vi "plcHMI_rev99.vi"() -> ()   [LabVIEW 2020]
doc: "ADS continuos synchronous write example using base blocks. \n\nThe client writes data synchronously and does wait for the respose from server."
uses:
  Agilent/AgilentTotalCluster.ctl
  Agilent/AgilentControl.ctl
  Agilent/Channel Config.ctl
  <vilib>/Platform/TimedLoop/XDataNode/timing_clust.ctl
  <vilib>/Platform/TimedLoop/XDataNode/nitl_modes.ctl
  <vilib>/Platform/TimedLoop/XDataNode/wakeup.ctl
  <userlib>/Beckhoff-LabVIEW-Interface/_DependsOn/With TypeResolving/Write Sync Single TypeResolved.vi
  <userlib>/Beckhoff-LabVIEW-Interface/_DependsOn/With TypeResolving/Read Sync Single TypeResolved.vi
  <vilib>/Platform/TimedLoop/XDataNode/XDataNode.xnode
  <vilib>/Platform/TimedLoop/XDataNode/XDNodeRunTimeDep.lvlib
panel:
  in  "Tab Control":T1(tab)
  out "error out":errorcluster
  in  "Symbol file path - MUST BE ENTERED\nLoad \"ADS Write AND Read Symbols REV X.X.xml\"":path
  out "bHasMached":bool
  out "Write Status":bool
  out "Read Status":bool
  in  "EXIT HMI":bool caption="STOP HMI\nEXIT HMI"
  out "Internal TwinCAT Handle ID Maps":dbl format="%#_12g"
  in  "802L TDK PSU Voltage Rating (abs(Volts))":i32=12000 min=1 max=50000
  in  "802L TDL PSU Peak Power (J/s)":i32=9000 min=1 max=50000
  in  "HVPS Model":u16(ring) items=["802L-12kV,9000J/s", "802L+50kV,9000J/s", "Other"]
  in  "Voltage Held by PSU":bool
  in  "Log Capacitor Voltage":bool
  in  "Log Temperature Data":bool
  out "Time Since Last Shot":string caption="Elapsed Time Text"
  in  "Duty Cycle":dbl
  in  "Current Control":bool
  out "Expected Voltage":i16
  in  "Dump":bool
  out "EOC":bool
  out "Maximum Test Number Reached":bool
  out "SCR Ready":bool
  in  "START":bool
  in  "STOP":bool
  in  "Hold":bool
  in  "Charge":bool
  in  "Shot":bool
  in  "HV Switch Mode":bool
  in  "CLEAR FAULT":bool
  in  "Manual/Auto":bool=TRUE
  out "Test Interval (Sec)":i32=15 min=0
  in  "Capacitance (uF)":sgl=1e-13 min=0 max=10000 format="%#_6f"
  in  "Target Charge Volt (V) - Min 1500V - TEMPORARY LIMIT 12kV":i32 min=-12000 max=12000 step=1
  out "Estimated Charge Time (seconds)":sgl
  in  "Hold Time Before Shot (seconds)":i16 max=1000
  in  "Max Number of Shots (Test intervals)":i32=1 min=1
  out "Shot Number":i16
  out "Charge Fault":bool=TRUE
  out "Discharge Fault":bool=TRUE
  out "Hold Fault":bool=TRUE
  out "Cap 1 Temp\nExceeded Fault":bool=TRUE
  out "Ambient Temp\nExceeded Fault":bool=TRUE
  out "PSU Fault":bool=TRUE
  out "Control Sys Fault":bool=TRUE
  out "test Running":bool
  out "Test State":string
  out "Cap 1 Voltage":i16
  out "Cap 1 Temperature":i16
  in  "Capacitor Voltage Data Log File Path (.xlsx)":path
  out "Load Temperature":i16
  out "Soft Dump Temp":i16
  out "Ambient Temp":i16
  out "Waveform Chart - Capacitor Voltage (Probe, abs(Volts))":dbl(graph)
  in  "Manual Charge Time (seconds)":sgl max=90
  in  "Reset Test Number":bool
  in  "Cap 1 Fault Temp (Cel)":i16 min=0 max=125
  in  "Capacitor Temperature Data Log File Path (.xlsx)":path
  out "Cap 1 Voltage (HVPS)":i16
  out "Capacitor Voltage":cluster{dbl, dbl}(graph)
  out "EOC":i16(graph)
  out "Soft Exception":bool
  out "PSU HV FB Fault":bool
  out "Charge FB Fault":bool
  out "Softdump FB Fault":bool
  out "SCR FB":i16(graph)
  in  "CH4 Vertical Units":string(combo)="V"
  in  "CH4 Vertical Units/div":dbl=2.0
  in  "Toggle Scope Scale":bool
  in  "CH1 Vertical Units/div":dbl=2.0
  in  "CH1 Vertical Units":string(combo)="V"
  in  "Horizontal Units":enum16{"us", "ms", "s"}(ring)
  in  "Horizontal Units/div":dbl=200.0
  out "Download":bool
  in  "Single":bool
  in  "Stop":bool
  out "Scope Trig":bool
  in  "Agilent Array":T2[](array[typedef])
  out "Process Step":i16
  in  "C:\\HVTest\\Local_Cap_Log_Scope (.xlsx)":path
  out "Stop Loops":bool
  # "CONFIGURATION"
  # "Press STOP HMI instead of\nLabView Abort Execution"
  # "PSU V Rating, Peak Power\nactive when OTHER\nis selected"
  # "INPUT VARIABLES - For TDK Lambda 802L\nMust be written to before START"
  # "FAULT STATUSES"
  # "Set to -1 for automated\nfull charge to setpoint"
  # "MANUAL CONTROLS"
  # "Does not record during \"wait\" and appends to data file. Must be named with .xlsx"
  # "HV Switch Configuration"
  # "Records during \"Test Running.\" Must be named with .xlsx"
  # "Control Sys Faults"
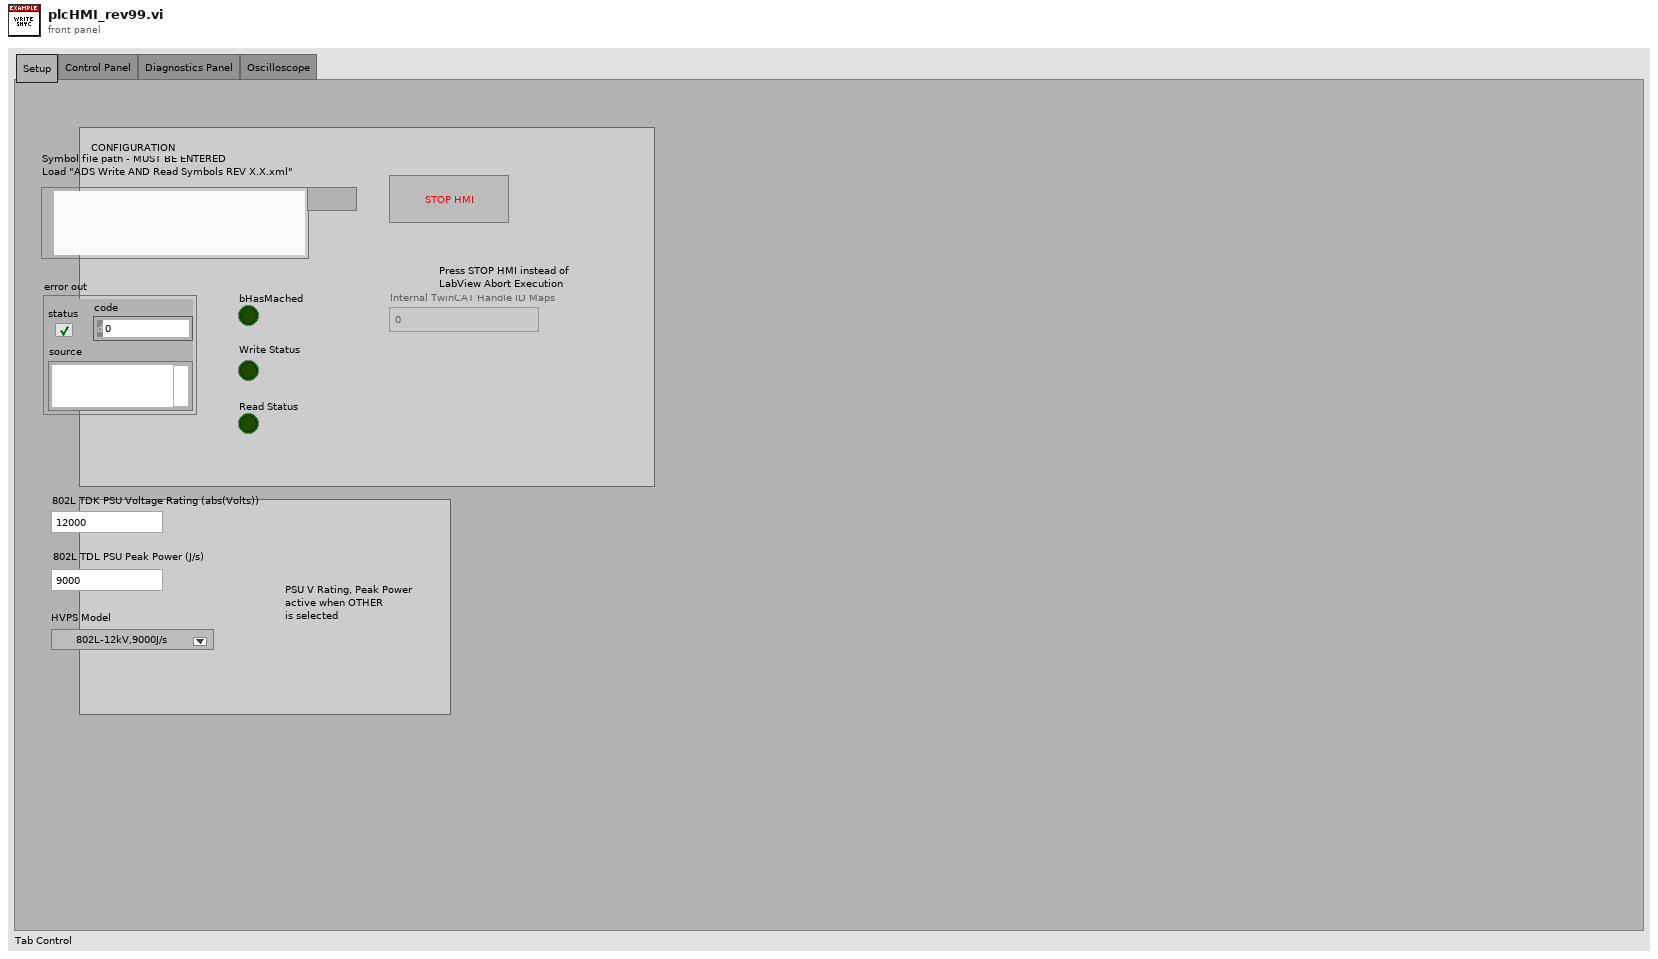
[diagram p1: front panel]
types:
  T1 = enum32{"Setup", "Control Panel", "Diagnostics Panel", "Oscilloscope"}
  T2 = typedef "AgilentTotalCluster.ctl" = cluster{"Agilent Graph":waveform(dbl)[], "Agilent Control":T3, "Agilent Setup Error":errorcluster, "Agilent Present":bool, "Enabled":bool}
  T3 = typedef "AgilentControl.ctl" = cluster{"Trig?":bool, "VISA session":refnum<visa-resource-name>, "Setup to Load":string, "Timeout (ms)":u32, "Desired Samp":enum32{"100", "250", "500", "1000", "2000", "5000", "10000", "20000", "50000", "100000", "200000", "500000", "1000000", "2000000", "4000000", "8000000"}, "Captured Samp":i32, "Desired Channels":T4[]}
  T4 = typedef "Channel Config.ctl" = cluster{"Chan Index":enum16{"Channel1", "Channel2", "Channel3", "Channel4", "MATH"}, "Name":string, "Samples":i32}
  T5 = typedef "XDNodeRunTimeDep.lvlib/timing_clust.ctl" = cluster{"Expected End [f-1]":u64, "Actual End [f-1]":u64, "Finished Late? [f-1]":bool, "Expected End [i-1]":u64, "Actual End [i-1]":u64, "Finished Late? [i-1]":bool, "Expected Start [i]":u64, "Actual Start [i]":u64, "Expected Start [f]":u64, "Actual Start [f]":u64, "Source Name":string, "Structure Name":string, "Period":i64, "Deadline":i64, "Offset":i64, "Start":i64, "Priority":i32, "Timeout":i32, "Mode":T6, "Wakeup Reason":T7, "Error":errorcluster, "Source Type":string, "Secondary Source Type":string, "Global End Time":u64, "Global Start Time":u64, "Frame Duration":u64, "Iteration Duration":u64, "Assigned CPU":i32, "I/O Scan Engine Mode":u32}
  T6 = typedef "XDNodeRunTimeDep.lvlib/nitl_modes.ctl" = enum32{"No Change", "Process missed periods, maintain original phase", "Discard missed periods, maintain original phase", "Process missed periods, ignore original phase", "Discard missed periods, ignore original phase"}
  T7 = typedef "XDNodeRunTimeDep.lvlib/wakeup.ctl" = enum32{"Normal", "Aborted", "Asynchronous wakeup", "Timing source error", "Timed loop error", "Timeout"}
  T8 = cluster{"Agilent Array[0]":T2, "Agilent Array[1]":T2, "Agilent Array[2]":T2, "Agilent Array[3]":T2, "Agilent Array[4]":T2, "Agilent Array[5]":T2, "Agilent Array[6]":T2, "Agilent Array[7]":T2, "Agilent Array[8]":T2}
  T9 = enum32{"100", "250", "500", "1000", "2000", "5000", "10000", "20000", "50000", "100000", "200000", "500000", "1000000", "2000000", "4000000", "8000000"}
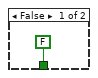
[diagram p2: hidden frame]
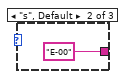
[diagram p5: hidden frame]
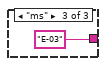
[diagram p6: hidden frame]
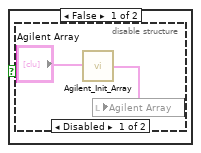
[diagram p7: hidden frame]
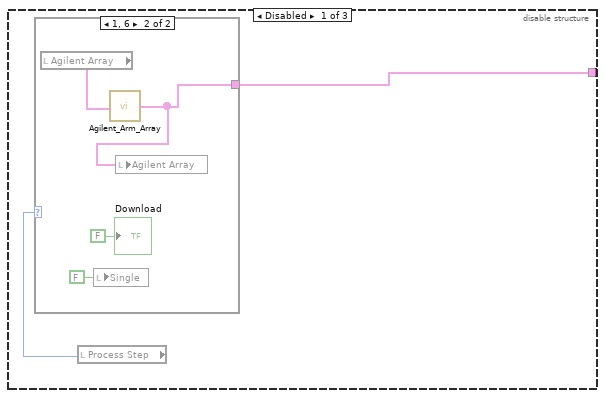
[diagram p11: hidden frame]
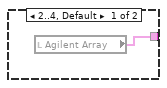
[diagram p12: hidden frame]
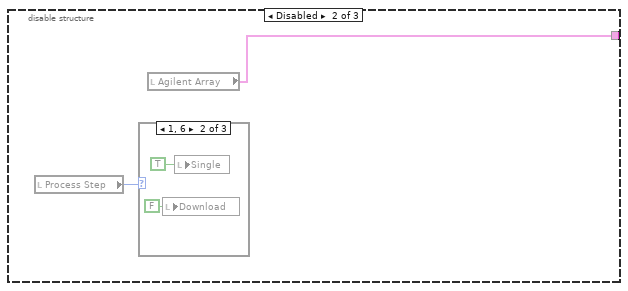
[diagram p13: hidden frame]
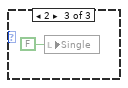
[diagram p15: hidden frame]
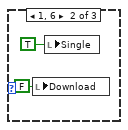
[diagram p17: hidden frame]
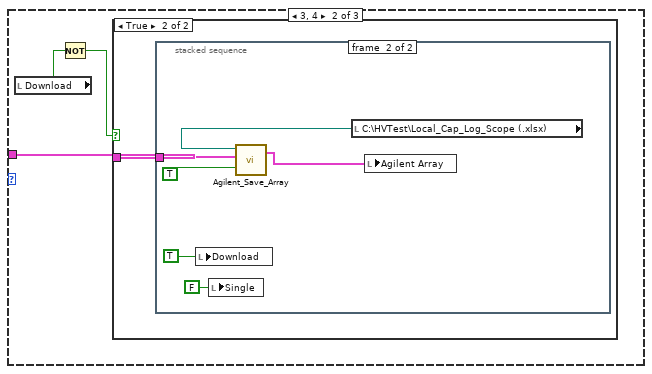
[diagram p19: hidden frame]
diagram:
  w85 = u16 17 items=["SyncLatest"=17, "AsyncLatest"=33] ("WriterMode")
  w154 = u16 33 items=["SyncLatest"=17, "AsyncLatest"=33] ("WriterMode")
  w194 = u16 33 items=["SyncLatest"=17, "AsyncLatest"=33] ("WriterMode")
  w213 = u16 33 items=["SyncLatest"=17, "AsyncLatest"=33] ("WriterMode")
  w232 = u16 33 items=["SyncLatest"=17, "AsyncLatest"=33] ("WriterMode")
  w251 = u16 33 items=["SyncLatest"=17, "AsyncLatest"=33] ("WriterMode")
  w270 = u16 17 items=["SyncLatest"=17, "AsyncLatest"=33] ("WriterMode")
  w289 = u16 17 items=["SyncLatest"=17, "AsyncLatest"=33] ("WriterMode")
  w308 = u16 17 items=["SyncLatest"=17, "AsyncLatest"=33] ("WriterMode")
  w327 = u16 17 items=["SyncLatest"=17, "AsyncLatest"=33] ("WriterMode")
  w346 = u16 17 items=["SyncLatest"=17, "AsyncLatest"=33] ("WriterMode")
  w365 = u16 17 items=["SyncLatest"=17, "AsyncLatest"=33] ("WriterMode")
  w384 = u16 17 items=["SyncLatest"=17, "AsyncLatest"=33] ("WriterMode")
  w399 = u16 17 items=["SyncLatest"=17, "AsyncLatest"=33] ("WriterMode")
  # "Variables/ Control"
  # "Documentation:\nCode separated vertically into two main sections - Write and read\nThey are further separated into BOOL and numeric\nThe OR gates wire all the error lines and the EXIT HMI button to a WHILE LOOP STOP\nThere current delay time on the routine is 100ms\nAll the AND gates connect the typecast resolve lines to the bHasMatched indicator\nThe second and third set of AND gates connect the write statuses to the Write Status indicator\nThe same is done for the read status indicator"
  # "WRITE NUMERICS"
  # "WRITE BOOLS"
  # "Select Symbol N"
  # "Read Initialization"
  # "Release \nTypeResolver"
  # "Release Writer"
  # "Send Request"
  # "Init \nTypeResolver"
  # "Init Writer"
  # "Select Symbol"
  # "Initialization"
  # "Call Release handle block\nat the end, when all nodes\nhave finished their execution"
  # "There must be only one release\nafter every init block.\nRelease block must be called\nalways at the end."
  # "Release"
  # "Symbol Interface"
  n1 = disable-structure shown="Enabled" {
    disable-tunnel: [w405 _] -> w403
    disable-tunnel: [w404 w407] -> w402
    frame Disabled {
      # "Using Symbol Interface"
      n2 = call <userlib>:"Symbol Interface.vi"() -> ("PortInfo"=w404:string, "error out"=w405:errorcluster)  [unwired: 14 in]
    }
    frame Enabled {
      # "Using Symbol File"
      n3 = Path To String(path="Symbol file path - MUST BE ENTERED\nLoad \"ADS Write AND Read Symbols REV X.X.xml\"") -> (string=w407:string)
    }
  }
  n4 = call <userlib>:"Init.vi"("XMLDescription"=w402, "error in (no error)"=w403) -> ("Handle"=w35:u32, "ReadGrpSymbols"=w18:string[], "WriteGrpSymbols"=w23:string[], "error out"=w2:errorcluster)  [unwired: 9 in, 1 out]
  n5 = Index Array(array=w23, index=0) -> (element=w13:string)
  n6 = Index Array(array=w23, index=20) -> (element=w22:string)
  n7 = Index Array(array=w23, index=19) -> (element=w28:string)
  n8 = Index Array(array=w23, index=13) -> (element=w3:string)
  n9 = Index Array(array=w23, index=9) -> (element=w252:string)
  n10 = Index Array(array=w23, index=11) -> (element=w214:string)
  n11 = Index Array(array=w23, index=10) -> (element=w233:string)
  n12 = Index Array(array=w23, index=12) -> (element=w195:string)
  n13 = Index Array(array=w23, index=17) -> (element=w36:string)
  n14 = Index Array(array=w23, index=18) -> (element=w29:string)
  n15 = Index Array(array=w23, index=7) -> (element=w271:string)
  n16 = Index Array(array=w23, index=2) -> (element=w366:string)
  n17 = Index Array(array=w23, index=3) -> (element=w347:string)
  n18 = Index Array(array=w23, index=5) -> (element=w309:string)
  n19 = Index Array(array=w23, index=4) -> (element=w328:string)
  n20 = Index Array(array=w23, index=6) -> (element=w290:string)
  n21 = Index Array(array=w23, index=1) -> (element=w385:string)
  n22 = Index Array(array=w23, index=15) -> (element=w6:string)
  n23 = Index Array(array=w23, index=8) -> (element=w84:string)
  n24 = Index Array(array=w23, index=14) -> (element=w155:string)
  n25 = Index Array(array=w23, index=16) -> (element=w8:string)
  n26 = call <userlib>:"Init Writer.vi"("Handle"=w35, "SymbolName"=w252, "WriterMode"=w251, "error constant"=w2) -> ("Handle"=w250:u32, "SymbolName"=w249:string, "WriterMode"=w248:u16, "WriteHandle"=w247:u32, "error IO"=w246:errorcluster)  [unwired: 7 in]
  n27 = call <userlib>:"Init Writer.vi"("Handle"=w35, "SymbolName"=w214, "WriterMode"=w213, "error constant"=w2) -> ("Handle"=w212:u32, "SymbolName"=w211:string, "WriterMode"=w210:u16, "WriteHandle"=w209:u32, "error IO"=w208:errorcluster)  [unwired: 7 in]
  n28 = call <userlib>:"Init Type.vi"("Handle"=w35, "SymbolName"=w252, "error in"=w2) -> ("Handle"=w245:u32, "TypeHdl"=w244:u32, "error IO"=w243:errorcluster)  [unwired: 7 in, 3 out]
  n29 = call <userlib>:"Init Writer.vi"("Handle"=w35, "SymbolName"=w233, "WriterMode"=w232, "error constant"=w2) -> ("Handle"=w231:u32, "SymbolName"=w230:string, "WriterMode"=w229:u16, "WriteHandle"=w228:u32, "error IO"=w227:errorcluster)  [unwired: 7 in]
  n30 = call <userlib>:"Init Type.vi"("Handle"=w35, "SymbolName"=w214, "error in"=w2) -> ("Handle"=w207:u32, "TypeHdl"=w206:u32, "error IO"=w205:errorcluster)  [unwired: 7 in, 3 out]
  n31 = call <userlib>:"Init Writer.vi"("Handle"=w35, "SymbolName"=w195, "WriterMode"=w194, "error constant"=w2) -> ("Handle"=w193:u32, "SymbolName"=w192:string, "WriterMode"=w191:u16, "WriteHandle"=w190:u32, "error IO"=w189:errorcluster)  [unwired: 7 in]
  n32 = call <userlib>:"Init Type.vi"("Handle"=w35, "SymbolName"=w233, "error in"=w2) -> ("Handle"=w226:u32, "TypeHdl"=w225:u32, "error IO"=w224:errorcluster)  [unwired: 7 in, 3 out]
  n33 = call <userlib>:"Init Type.vi"("Handle"=w35, "SymbolName"=w195, "error in"=w2) -> ("Handle"=w188:u32, "TypeHdl"=w187:u32, "error IO"=w186:errorcluster)  [unwired: 7 in, 3 out]
  n34 = call <userlib>:"Init Writer.vi"("Handle"=w35, "SymbolName"=w271, "WriterMode"=w270, "error constant"=w2) -> ("Handle"=w269:u32, "SymbolName"=w268:string, "WriterMode"=w267:u16, "WriteHandle"=w266:u32, "error IO"=w265:errorcluster)  [unwired: 7 in]
  n35 = call <userlib>:"Init Writer.vi"("Handle"=w35, "SymbolName"=w366, "WriterMode"=w365, "error constant"=w2) -> ("Handle"=w361:u32, "SymbolName"=w360:string, "WriterMode"=w359:u16, "WriteHandle"=w357:u32, "error IO"=w358:errorcluster)  [unwired: 7 in]
  n36 = call <userlib>:"Init Writer.vi"("Handle"=w35, "SymbolName"=w347, "WriterMode"=w346, "error constant"=w2) -> ("Handle"=w345:u32, "SymbolName"=w344:string, "WriterMode"=w343:u16, "WriteHandle"=w342:u32, "error IO"=w341:errorcluster)  [unwired: 7 in]
  n37 = call <userlib>:"Init Writer.vi"("Handle"=w35, "SymbolName"=w309, "WriterMode"=w308, "error constant"=w2) -> ("Handle"=w307:u32, "SymbolName"=w306:string, "WriterMode"=w305:u16, "WriteHandle"=w304:u32, "error IO"=w303:errorcluster)  [unwired: 7 in]
  n38 = call <userlib>:"Init Type.vi"("Handle"=w35, "SymbolName"=w271, "error in"=w2) -> ("Handle"=w264:u32, "TypeHdl"=w263:u32, "error IO"=w262:errorcluster)  [unwired: 7 in, 3 out]
  n39 = call <userlib>:"Init Type.vi"("Handle"=w35, "SymbolName"=w366, "error in"=w2) -> ("Handle"=w350:u32, "TypeHdl"=w349:u32, "error IO"=w348:errorcluster)  [unwired: 7 in, 3 out]
  n40 = call <userlib>:"Init Type.vi"("Handle"=w35, "SymbolName"=w347, "error in"=w2) -> ("Handle"=w340:u32, "TypeHdl"=w339:u32, "error IO"=w338:errorcluster)  [unwired: 7 in, 3 out]
  n41 = call <userlib>:"Init Writer.vi"("Handle"=w35, "SymbolName"=w328, "WriterMode"=w327, "error constant"=w2) -> ("Handle"=w326:u32, "SymbolName"=w325:string, "WriterMode"=w324:u16, "WriteHandle"=w323:u32, "error IO"=w322:errorcluster)  [unwired: 7 in]
  n42 = call <userlib>:"Init Type.vi"("Handle"=w35, "SymbolName"=w309, "error in"=w2) -> ("Handle"=w302:u32, "TypeHdl"=w301:u32, "error IO"=w300:errorcluster)  [unwired: 7 in, 3 out]
  n43 = call <userlib>:"Init Writer.vi"("Handle"=w35, "SymbolName"=w290, "WriterMode"=w289, "error constant"=w2) -> ("Handle"=w288:u32, "SymbolName"=w287:string, "WriterMode"=w286:u16, "WriteHandle"=w285:u32, "error IO"=w284:errorcluster)  [unwired: 7 in]
  n44 = call <userlib>:"Init Type.vi"("Handle"=w35, "SymbolName"=w328, "error in"=w2) -> ("Handle"=w321:u32, "TypeHdl"=w320:u32, "error IO"=w319:errorcluster)  [unwired: 7 in, 3 out]
  n45 = call <userlib>:"Init Type.vi"("Handle"=w35, "SymbolName"=w290, "error in"=w2) -> ("Handle"=w283:u32, "TypeHdl"=w282:u32, "error IO"=w281:errorcluster)  [unwired: 7 in, 3 out]
  n46 = call <userlib>:"Init Writer.vi"("Handle"=w35, "SymbolName"=w385, "WriterMode"=w384, "error constant"=w2) -> ("Handle"=w383:u32, "SymbolName"=w382:string, "WriterMode"=w381:u16, "WriteHandle"=w380:u32, "error IO"=w379:errorcluster)  [unwired: 7 in]
  n47 = call <userlib>:"Init Type.vi"("Handle"=w35, "SymbolName"=w385, "error in"=w2) -> ("Handle"=w378:u32, "TypeHdl"=w377:u32, "error IO"=w376:errorcluster)  [unwired: 7 in, 3 out]
  n48 = call <userlib>:"Init Writer.vi"("Handle"=w35, "SymbolName"=w13, "WriterMode"=w399, "error constant"=w2) -> ("Handle"=w398:u32, "SymbolName"=w397:string, "WriterMode"=w396:u16, "WriteHandle"=w395:u32, "error IO"=w394:errorcluster)  [unwired: 7 in]
  n49 = call <userlib>:"Init Type.vi"("Handle"=w35, "SymbolName"=w13, "error in"=w2) -> ("Handle"=w393:u32, "TypeHdl"=w392:u32, "error IO"=w387:errorcluster)  [unwired: 7 in, 3 out]
  n50 = call <userlib>:"Init Writer.vi"("Handle"=w35, "SymbolName"=w155, "WriterMode"=w154, "error constant"=w2) -> ("Handle"=w150:u32, "SymbolName"=w149:string, "WriterMode"=w148:u16, "WriteHandle"=w140:u32, "error IO"=w147:errorcluster)  [unwired: 7 in]
  n51 = call <userlib>:"Init Type.vi"("Handle"=w35, "SymbolName"=w155, "error in"=w2) -> ("Handle"=w145:u32, "TypeHdl"=w143:u32, "error IO"=w144:errorcluster)  [unwired: 7 in, 3 out]
  n52 = Index Array(array=w18, index=2) -> (element=w136:string)
  n53 = Index Array(array=w18, index=4) -> (element=w132:string)
  n54 = call <userlib>:"Init Writer.vi"("Handle"=w35, "SymbolName"=w84, "WriterMode"=w85, "error constant"=w2) -> ("Handle"=w83:u32, "SymbolName"=w82:string, "WriterMode"=w81:u16, "WriteHandle"=w80:u32, "error IO"=w79:errorcluster)  [unwired: 7 in]
  n55 = Index Array(array=w18, index=1) -> (element=w172:string)
  n56 = Index Array(array=w18, index=21) -> (element=w50:string)
  n57 = Index Array(array=w18, index=22) -> (element=w47:string)
  n58 = call <userlib>:"Init Type.vi"("Handle"=w35, "SymbolName"=w84, "error in"=w2) -> ("Handle"=w78:u32, "TypeHdl"=w77:u32, "error IO"=w76:errorcluster)  [unwired: 7 in, 3 out]
  n59 = Index Array(array=w18, index=0) -> (element=w171:string)
  n60 = Index Array(array=w18, index=3) -> (element=w133:string)
  n61 = Index Array(array=w18, index=20) -> (element=w55:string)
  n62 = Index Array(array=w18, index=23) -> (element=w46:string)
  n63 = Index Array(array=w18, index=16) -> (element=w138:string)
  n64 = Index Array(array=w18, index=24) -> (element=w44:string)
  n65 = Index Array(array=w18, index=11) -> (element=w160:string)
  n66 = Index Array(array=w18, index=10) -> (element=w161:string)
  n67 = Index Array(array=w18, index=17) -> (element=w58:string)
  n68 = Index Array(array=w18, index=18) -> (element=w57:string)
  n69 = Index Array(array=w18, index=13) -> (element=w158:string)
  n70 = Index Array(array=w18, index=12) -> (element=w159:string)
  n71 = Index Array(array=w18, index=15) -> (element=w156:string)
  n72 = Index Array(array=w18, index=19) -> (element=w56:string)
  n73 = Index Array(array=w18, index=26) -> (element=w17:string)
  n74 = Index Array(array=w18, index=5) -> (element=w69:string)
  n75 = Index Array(array=w18, index=6) -> (element=w126:string)
  n76 = Index Array(array=w18, index=9) -> (element=w170:string)
  n77 = Index Array(array=w18, index=14) -> (element=w157:string)
  n78 = Index Array(array=w18, index=8) -> (element=w128:string)
  n79 = Index Array(array=w18, index=25) -> (element=w33:string)
  n80 = Index Array(array=w18, index=7) -> (element=w127:string)
  n81 = node-c288(i64 100 ("Period")) -> (w93:T5)  [unwired: 2 in]
  n82 = timed-loop {
    tunnel: w398 -> [w700]
    tunnel: w397 -> [w699]
    tunnel: w396 -> [w698]
    tunnel: w395 -> [w697]
    tunnel: w393 -> [w929]
    tunnel: w392 -> [w928]
    tunnel: [w695] -> w391
    tunnel: [w694] -> w390
    tunnel: [w927] -> w389
    tunnel: [w926] -> w388
    tunnel: w383 -> [w924]
    tunnel: w382 -> [w923]
    tunnel: w381 -> [w922]
    tunnel: w380 -> [w921]
    tunnel: w378 -> [w919]
    tunnel: w377 -> [w918]
    tunnel: [w916] -> w374
    tunnel: [w915] -> w373
    tunnel: [w914] -> w371
    tunnel: [w913] -> w370
    tunnel: w361 -> [w912]
    tunnel: w360 -> [w911]
    tunnel: w359 -> [w910]
    tunnel: w357 -> [w908]
    tunnel: [w907] -> w356
    tunnel: [w906] -> w355
    tunnel: [w905] -> w352
    tunnel: [w904] -> w351
    tunnel: w350 -> [w903]
    tunnel: w349 -> [w902]
    tunnel: w345 -> [w900]
    tunnel: w344 -> [w899]
    tunnel: w343 -> [w898]
    tunnel: w342 -> [w897]
    tunnel: w340 -> [w895]
    tunnel: w339 -> [w894]
    tunnel: [w892] -> w336
    tunnel: [w891] -> w335
    tunnel: [w890] -> w333
    tunnel: [w889] -> w332
    tunnel: w326 -> [w888]
    tunnel: w325 -> [w887]
    tunnel: w324 -> [w886]
    tunnel: w323 -> [w885]
    tunnel: w321 -> [w883]
    tunnel: w320 -> [w882]
    tunnel: [w880] -> w317
    tunnel: [w879] -> w316
    tunnel: [w878] -> w314
    tunnel: [w877] -> w313
    tunnel: w307 -> [w876]
    tunnel: w306 -> [w875]
    tunnel: w305 -> [w874]
    tunnel: w304 -> [w873]
    tunnel: w302 -> [w871]
    tunnel: w301 -> [w870]
    tunnel: [w868] -> w298
    tunnel: [w867] -> w297
    tunnel: [w866] -> w295
    tunnel: [w865] -> w294
    tunnel: w288 -> [w864]
    tunnel: w287 -> [w863]
    tunnel: w286 -> [w862]
    tunnel: w285 -> [w861]
    tunnel: w283 -> [w859]
    tunnel: w282 -> [w858]
    tunnel: [w856] -> w279
    tunnel: [w855] -> w278
    tunnel: [w854] -> w276
    tunnel: [w853] -> w275
    tunnel: w269 -> [w852]
    tunnel: w268 -> [w851]
    tunnel: w267 -> [w850]
    tunnel: w266 -> [w849]
    tunnel: w264 -> [w847]
    tunnel: w263 -> [w846]
    tunnel: [w844] -> w260
    tunnel: [w843] -> w259
    tunnel: [w842] -> w257
    tunnel: [w841] -> w256
    tunnel: w250 -> [w840]
    tunnel: w249 -> [w839]
    tunnel: w248 -> [w838]
    tunnel: w247 -> [w837]
    tunnel: w245 -> [w835]
    tunnel: w244 -> [w834]
    tunnel: [w832] -> w241
    tunnel: [w831] -> w240
    tunnel: [w830] -> w238
    tunnel: [w829] -> w237
    tunnel: w231 -> [w828]
    tunnel: w230 -> [w827]
    tunnel: w229 -> [w826]
    tunnel: w228 -> [w825]
    tunnel: w226 -> [w823]
    tunnel: w225 -> [w822]
    tunnel: [w820] -> w222
    tunnel: [w819] -> w221
    tunnel: [w818] -> w219
    tunnel: [w817] -> w218
    tunnel: w212 -> [w816]
    tunnel: w211 -> [w815]
    tunnel: w210 -> [w814]
    tunnel: w209 -> [w813]
    tunnel: w207 -> [w811]
    tunnel: w206 -> [w810]
    tunnel: [w808] -> w203
    tunnel: [w807] -> w202
    tunnel: [w806] -> w200
    tunnel: [w805] -> w199
    tunnel: w193 -> [w804]
    tunnel: w192 -> [w803]
    tunnel: w191 -> [w802]
    tunnel: w190 -> [w801]
    tunnel: w188 -> [w799]
    tunnel: w187 -> [w798]
    tunnel: [w796] -> w184
    tunnel: [w795] -> w183
    tunnel: [w794] -> w181
    tunnel: [w793] -> w180
    tunnel: w172 -> [w792]
    tunnel: w171 -> [w791]
    tunnel: w170 -> [w790]
    tunnel: [w789] -> w121
    tunnel: w161 -> [w788]
    tunnel: w160 -> [w787]
    tunnel: w159 -> [w786]
    tunnel: w158 -> [w785]
    tunnel: w157 -> [w784]
    tunnel: w156 -> [w783]
    tunnel: [w782] -> w90
    tunnel: [w781] -> w120
    tunnel: [w780] -> w119
    tunnel: [w779] -> w118
    tunnel: [w778] -> w117
    tunnel: [w723] -> w116
    tunnel: [w721] -> w115
    shift-right: [w626] -> w401
    shift-left: w394 -> [w696]
    shift-right: [w625] -> w400
    shift-left: w387 -> [w925]
    shift-right: [w623] -> w372
    shift-left: w379 -> [w920]
    shift-right: [w622] -> w369
    shift-left: w376 -> [w917]
    shift-right: [w620] -> w354
    shift-left: w358 -> [w909]
    shift-right: [w619] -> w353
    shift-left: w348 -> [w901]
    shift-right: [w617] -> w334
    shift-left: w341 -> [w896]
    shift-right: [w616] -> w331
    shift-left: w338 -> [w893]
    shift-right: [w614] -> w315
    shift-left: w322 -> [w884]
    shift-right: [w613] -> w312
    shift-left: w319 -> [w881]
    shift-right: [w611] -> w296
    shift-left: w303 -> [w872]
    shift-right: [w610] -> w293
    shift-left: w300 -> [w869]
    shift-right: [w608] -> w277
    shift-left: w284 -> [w860]
    shift-right: [w607] -> w274
    shift-left: w281 -> [w857]
    shift-right: [w605] -> w258
    shift-left: w265 -> [w848]
    shift-right: [w604] -> w255
    shift-left: w262 -> [w845]
    shift-right: [w603] -> w239
    shift-left: w246 -> [w836]
    shift-right: [w602] -> w236
    shift-left: w243 -> [w833]
    shift-right: [w600] -> w220
    shift-left: w227 -> [w824]
    shift-right: [w599] -> w217
    shift-left: w224 -> [w821]
    shift-right: [w597] -> w201
    shift-left: w208 -> [w812]
    shift-right: [w596] -> w198
    shift-left: w205 -> [w809]
    shift-right: [w594] -> w182
    shift-left: w189 -> [w800]
    shift-right: [w593] -> w179
    shift-left: w186 -> [w797]
    tunnel: w150 -> [w763]
    tunnel: w149 -> [w762]
    tunnel: w148 -> [w761]
    tunnel: [w759] -> w12
    tunnel: [w758] -> w146
    tunnel: w145 -> [w757]
    tunnel: w143 -> [w755]
    tunnel: [w754] -> w142
    tunnel: [w753] -> w141
    tunnel: w140 -> [w752]
    tunnel: w138 -> [w751]
    tunnel: [w722] -> w114
    tunnel: [w745] -> w123
    tunnel: w2 -> [w744]
    tunnel: [w742] -> w122
    tunnel: w136 -> [w741]
    tunnel: w133 -> [w737]
    tunnel: w132 -> [w736]
    tunnel: [w727] -> w124
    tunnel: [w726] -> w125
    tunnel: w128 -> [w720]
    tunnel: w127 -> [w719]
    tunnel: w126 -> [w718]
    tunnel: [w705] -> w66
    tunnel: [w704] -> w65
    tunnel: [w703] -> w64
    timing: w93 -> [_]
    timing-out: [_] -> w92
    tunnel: w35 -> [w693]
    tunnel: [w591] -> w68
    tunnel: w83 -> [w586]
    tunnel: w82 -> [w585]
    tunnel: w81 -> [w584]
    tunnel: w80 -> [w583]
    tunnel: w78 -> [w581]
    tunnel: w77 -> [w580]
    tunnel: [w577] -> w75
    tunnel: [w576] -> w74
    tunnel: [w575] -> w73
    tunnel: [w574] -> w72
    tunnel: [w567] -> w67
    tunnel: w69 -> [w563]
    tunnel: [w562] -> w63
    tunnel: w58 -> [w559]
    tunnel: w57 -> [w554]
    tunnel: w56 -> [w553]
    tunnel: w55 -> [w552]
    tunnel: [w549] -> w54
    tunnel: [w547] -> w53
    tunnel: [w542] -> w52
    tunnel: [w541] -> w39
    tunnel: w50 -> [w539]
    tunnel: w47 -> [w514]
    tunnel: w46 -> [w513]
    tunnel: w44 -> [w506]
    tunnel: [w502] -> w43
    tunnel: [w501] -> w42
    tunnel: [w500] -> w41
    tunnel: [w499] -> w40
    tunnel: w36 -> [w498]
    tunnel: w35 -> [w417]
    tunnel: w2 -> [w497]
    tunnel: [w494] -> w27
    tunnel: [w493] -> _
    tunnel: w33 -> [w489]
    tunnel: [w485] -> w32
    tunnel: w29 -> [w484]
    tunnel: w28 -> [w483]
    tunnel: w2 -> [w461]
    tunnel: [w478] -> w26
    tunnel: [w477] -> w25
    tunnel: w22 -> [w465]
    tunnel: [w460] -> w21
    tunnel: w17 -> [w447]
    tunnel: [w445] -> w16
    shift-right: [w443] -> w15
    shift-left: w147 -> [w760]
    shift-right: [w442] -> w14
    shift-left: w144 -> [w756]
    tunnel: w2 -> [w435]
    tunnel: [w432] -> w7
    shift-right: [w440] -> w10
    shift-left: w79 -> [w582]
    shift-right: [w439] -> w9
    shift-left: w76 -> [w579]
    tunnel: w8 -> [w434]
    tunnel: w6 -> [w427]
    tunnel: w2 -> [w426]
    tunnel: [w425] -> w5
    tunnel: w3 -> [w418]
    tunnel: w2 -> [w416]
    tunnel: [w415] -> w1
    stop <- w410 stop-if-true
    # "Stop Loop on Error (OR gates)"
    # "Error Stop Loop AND"
    # "Typecast Match AND"
    # "Write Status AND"
    # "READ BOOLS"
    # "READ NUMERICS"
    # "STOP HMI via error or EXIT button"
    # "Check Read status and\nthen convert Variant \nto LabVIEW type (AND gates)"
    # "Sync Read Single"
    n83 = node-c288() -> (w592:errorcluster)  [unwired: 1 in]
    n84 = disable-structure shown="Enabled" {
      frame Enabled {
        n85 = flat-sequence {
          tunnel: [w1061] -> w1005
          tunnel: w1005 -> [w1080]
          frame #0 {
            n86 = disable-structure shown="Enabled" {
              frame Enabled {
                n87 = feedback #1(TRUE) -> (w1007:bool)
                n88 = And(x=TRUE, y=w1007) -> (x .and. y?=w1010:bool)
                n89 = case shown="True" w1010 {
                  tunnel: [FALSE FALSE] -> w1008
                  frame False {
                  }
                  frame True {
                    n90 = local read "Agilent Array"() -> (w1013:T2[])
                    n91 = call "Agilent_Init_Array.vi"("Agilent Array In"=w1013) -> ("Agilent Array Out"=w1014:T2[])
                    n92 = call "Agilent_Arm_Array.vi"("Agilent Array In"=w1014) -> ("Agilent Array Out"=w1012:T2[])
                    n93 = local write "Agilent Array"(w1012) -> ()
                  }
                }
                n94 = feedback-in #1(w1008) -> ()
              }
              frame Disabled {
              }
            }
          }
          frame #1 {
            n95 = case shown="True" "Toggle Scope Scale" {
              frame False {
              }
              frame True {
                n96 = Number To Decimal String(number="CH4 Vertical Units/div") -> (decimal integer string=w1020:string)  [unwired: 1 in]
                n97 = Number To Decimal String(number="Horizontal Units/div") -> (decimal integer string=w1028:string)  [unwired: 1 in]
                n98 = Number To Decimal String(number="CH1 Vertical Units/div") -> (decimal integer string=w1026:string)  [unwired: 1 in]
                n99 = case shown="\"us\"" "Horizontal Units" {
                  tunnel: ["E-06" "E-00" "E-03"] -> w1037
                  frame "us" {
                  }
                  frame "s", Default {
                  }
                  frame "ms" {
                  }
                }
                n100 = Concatenate Strings(":CHAN4:SCAL " ("write buffer"), w1020, "CH4 Vertical Units") -> (w1019:string)
                n101 = Concatenate Strings(":CHAN1:SCAL " ("write buffer"), w1026, "CH1 Vertical Units") -> (w1033:string)
                n102 = Concatenate Strings(":TIM:SCAL " ("write buffer"), w1028, w1037) -> (w1036:string)
                n103 = VISA Open(VISA resource name=refnum<visa-resource-name> "HV_Test_Scope") -> (VISA resource name=w1031:refnum<visa-resource-name>, error out=w1032:errorcluster)  [unwired: 4 in]
                n104 = VISA Write(VISA resource name=w1031, write buffer=w1036, error in (no error)=w1032) -> (VISA resource name out=w1040:refnum<visa-resource-name>, error out=w1039:errorcluster)  [unwired: 1 out]
                n105 = VISA Write(VISA resource name=w1040, write buffer=w1033, error in (no error)=w1039) -> (VISA resource name out=w1025:refnum<visa-resource-name>, error out=w1023:errorcluster)  [unwired: 1 out]
                n106 = VISA Write(VISA resource name=w1025, write buffer=w1019, error in (no error)=w1023) -> (VISA resource name out=w1024:refnum<visa-resource-name>, error out=w1022:errorcluster)  [unwired: 1 out]
                n107 = VISA Close(VISA resource name=w1024, error in (no error)=w1022) -> ()  [unwired: 1 out]
              }
            }
          }
          frame #2 {
            n108 = disable-structure shown="Enabled" {
              frame Enabled {
                n109 = case shown="True" "Stop" {
                  frame False {
                    n110 = disable-structure shown="Disabled" {
                      frame Disabled {
                        n111 = call "Agilent_Init_Array.vi"("Agilent Array In"="Agilent Array") -> ("Agilent Array Out"=w1047:T2[])
                        n112 = local write "Agilent Array"(w1047) -> ()
                      }
                      frame Enabled {
                      }
                    }
                  }
                  frame True {
                    n113 = VISA Open(VISA resource name=refnum<visa-resource-name> "HV_Test_Scope") -> (VISA resource name=w1053:refnum<visa-resource-name>, error out=w1054:errorcluster)  [unwired: 4 in]
                    n114 = VISA Write(VISA resource name=w1053, write buffer=":STOP", error in (no error)=w1054) -> (VISA resource name out=w1051:refnum<visa-resource-name>, error out=w1052:errorcluster)  [unwired: 1 out]
                    n115 = VISA Close(VISA resource name=w1051, error in (no error)=w1052) -> ()  [unwired: 1 out]
                  }
                }
              }
              frame Disabled {
              }
            }
            n116 = case shown="True" "Single" {
              frame False {
              }
              frame True {
                n117 = VISA Open(VISA resource name=refnum<visa-resource-name> "HV_Test_Scope") -> (VISA resource name=w1059:refnum<visa-resource-name>, error out=w1060:errorcluster)  [unwired: 4 in]
                n118 = VISA Write(VISA resource name=w1059, write buffer=":SINGLE", error in (no error)=w1060) -> (VISA resource name out=w1057:refnum<visa-resource-name>, error out=w1058:errorcluster)  [unwired: 1 out]
                n119 = VISA Close(VISA resource name=w1057, error in (no error)=w1058) -> ()  [unwired: 1 out]
              }
            }
          }
          frame #3 {
            n120 = disable-structure shown="Enabled" {
              disable-tunnel: [w1063 w1070 w1075] -> w1061
              frame Disabled {
                n121 = local read "Process Step"() -> (w1062:i16)
                n122 = case shown="1, 6" w1062 {
                  tunnel: [w1064 w1068] -> w1063
                  frame 2..4, Default {
                    n123 = local read "Agilent Array"() -> (w1064:T2[])
                  }
                  frame 1, 6 {
                    n124 = local read "Agilent Array"() -> (w1065:T2[])
                    n125 = local write "Single"(FALSE ("Single")) -> ()
                    n126 = call "Agilent_Arm_Array.vi"("Agilent Array In"=w1065) -> ("Agilent Array Out"=w1068:T2[])
                    n127 = local write "Agilent Array"(w1068) -> ()
                    "Download" <- FALSE ("Downloading")
                  }
                }
              }
              frame Disabled {
                n128 = local read "Process Step"() -> (w1069:i16)
                n129 = case shown="1, 6" w1069 {
                  frame 0, Default {
                  }
                  frame 1, 6 {
                    n130 = local write "Download"(FALSE ("Download")) -> ()
                    n131 = local write "Single"(TRUE ("Single")) -> ()
                  }
                  frame 2 {
                    n132 = local write "Single"(FALSE ("Single")) -> ()
                  }
                }
                n133 = local read "Agilent Array"() -> (w1070:T2[])
              }
              frame Enabled {
                n134 = local read "Process Step"() -> (w1074:i16)
                n135 = case shown="2, 7" w1074 {
                  frame 0, Default {
                  }
                  frame 1, 6 {
                    n136 = local write "Download"(FALSE ("Download")) -> ()
                    n137 = local write "Single"(TRUE ("Single")) -> ()
                  }
                  frame 2, 7 {
                    n138 = local write "Single"(FALSE ("Single")) -> ()
                  }
                }
                n139 = local read "Agilent Array"() -> (w1075:T2[])
              }
            }
          }
          frame #4 {
            n140 = local read "Process Step"() -> (w1079:i16)
            n141 = case shown="0" w1079 {
              tunnel: w1080 -> [_ w1083 w1096]
              frame Default {
              }
              frame 3, 4 {
                n142 = local read "Download"() -> (w1082:bool)
                n143 = Not(x=w1082) -> (.not. x?=w1081:bool)
                n144 = case shown="True" w1081 {
                  tunnel: w1083 -> [_ w1084]
                  frame False {
                  }
                  frame True {
                    n145 = stacked-sequence {
                      tunnel: w1084 -> [_ w1094]
                      frame #0 {
                        n146 = local read "Agilent Array"() -> (w1088:T2[])
                        n147 = Array To Cluster(array=w1088) -> (cluster=w1087:T8)
                        n148 = Unbundle By Name(w1087) -> ("Agilent Array[0].Agilent Control.Desired Samp"=w1085:T9)
                        n149 = call "GF_SetRecordLengthProperly.vi"("Num Samples"=w1085, "VISA resource name"=refnum<visa-resource-name> "HV_Test_Scope") -> ()  [unwired: 1 in, 2 out]
                      }
                      frame #1 {
                        n150 = local write "Download"(TRUE ("Downloading")) -> ()
                        n151 = local write "Single"(FALSE ("Single")) -> ()
                        n152 = local read "C:\\HVTest\\Local_Cap_Log_Scope (.xlsx)"() -> (w1089:path)
                        n153 = call "Agilent_Save_Array.vi"("Agilent Download"=TRUE, "Agilent Array In"=w1094, "File Path"=w1089) -> ("Agilent Array Out"=w1092:T2[])  [unwired: 1 in, 1 out]
                        n154 = local write "Agilent Array"(w1092) -> ()
                      }
                    }
                  }
                }
              }
              frame 0 {
                n155 = local read "Maximum Test Number Reached"() -> (w1095:bool)
                n156 = case shown="True" w1095 {
                  tunnel: w1096 -> [_ w1099]
                  frame False {
                  }
                  frame True {
                    n157 = local read "Download"() -> (w1098:bool)
                    n158 = Not(x=w1098) -> (.not. x?=w1097:bool)
                    n159 = case shown="True" w1097 {
                      tunnel: w1099 -> [_ w1100]
                      frame False {
                      }
                      frame True {
                        n160 = stacked-sequence {
                          tunnel: w1100 -> [_ w1110]
                          frame #0 {
                            n161 = local read "Agilent Array"() -> (w1104:T2[])
                            n162 = Array To Cluster(array=w1104) -> (cluster=w1103:T8)
                            n163 = Unbundle By Name(w1103) -> ("Agilent Array[0].Agilent Control.Desired Samp"=w1101:T9)
                            n164 = call "GF_SetRecordLengthProperly.vi"("Num Samples"=w1101, "VISA resource name"=refnum<visa-resource-name> "HV_Test_Scope") -> ()  [unwired: 1 in, 2 out]
                          }
                          frame #1 {
                            n165 = local write "Download"(TRUE ("Downloading")) -> ()
                            n166 = local write "Single"(FALSE ("Single")) -> ()
                            n167 = call "Agilent_Save_Array.vi"("Agilent Download"=TRUE, "Agilent Array In"=w1110, "File Path"="C:\\HVTest\\Local_Cap_Log_Scope (.xlsx)") -> ("Agilent Array Out"=w1108:T2[])  [unwired: 1 in, 1 out]
                            n168 = local write "Agilent Array"(w1108) -> ()
                          }
                        }
                      }
                    }
                  }
                }
              }
            }
          }
        }
      }
      frame Disabled {
      }
    }
    n169 = To Long Integer(number="Max Number of Shots (Test intervals)") -> (32bit integer=w421:i32)
    n170 = To Variant(anything=w421) -> (Variant=w420:variant)
    n171 = case shown="0, Default" "HVPS Model" {
      tunnel: ["802L TDK PSU Voltage Rating (abs(Volts))" 12000 50000] -> w701
      tunnel: ["802L TDL PSU Peak Power (J/s)" 9000 9000] -> w724
      frame 2 {
      }
      frame 0, Default {
      }
      frame 1 {
      }
    }
    n172 = call-poly <userlib>:"Write TypeResolved.vi"("Handle"=w417, "SymbolName"=w418, "WData"=w420, "error constant"=w416) -> ("Write Status?"=w412:bool, "Has Matched?"=w413:bool, "error out"=w415:errorcluster)  [unwired: 8 in, 1 out]
    n173 = To Single Precision Float(number="Manual Charge Time (seconds)") -> (single precision float=w429:sgl)
    n174 = To Variant(anything=w429) -> (Variant=w428:variant)
    n175 = flat-sequence {
      tunnel: w757 -> [w1208]
      tunnel: w755 -> [w1209]
      tunnel: w756 -> [w1210]
      tunnel: [w1210] -> w767
      tunnel: [w1209] -> w766
      tunnel: [w1208] -> w765
      tunnel: [w1207] -> w764
      tunnel: w724 -> [w1206]
      tunnel: [w1213] -> w442
      tunnel: [w1216] -> w753
      tunnel: [w1215] -> w754
      tunnel: [w1214] -> w444
      tunnel: w767 -> [w1219]
      tunnel: w766 -> [w1218]
      tunnel: w765 -> [w1217]
      tunnel: w764 -> [w1212]
      tunnel: [w1211] -> w650
      frame #0 {
        # "Write Data"
        n176 = To Long Integer(number=w1206) -> (32bit integer=w1205:i32)
        n177 = To Variant(anything=w1205) -> (Variant=w1207:variant)
      }
      frame #1 {
        # "Resolve To TC"
        n178 = call <userlib>:"Resolve To TC Type.vi"("Handle"=w1217, "TypHdl"=w1218, "WData"=w1212, "error in"=w1219) -> ("Handle"=w1215:u32, "TypHdl"=w1216:u32, "bHasMatched"=w1211:bool, "ADSWData"=w1214:variant, "error out"=w1213:errorcluster)  [unwired: 7 in]
      }
    }
    n179 = flat-sequence {
      tunnel: w835 -> [w1358]
      tunnel: w834 -> [w1359]
      tunnel: w833 -> [w1360]
      tunnel: [w1360] -> w969
      tunnel: [w1359] -> w968
      tunnel: [w1358] -> w967
      tunnel: [w1357] -> w966
      tunnel: [w1363] -> w602
      tunnel: [w1366] -> w829
      tunnel: [w1365] -> w830
      tunnel: [w1364] -> w771
      tunnel: w969 -> [w1369]
      tunnel: w968 -> [w1368]
      tunnel: w967 -> [w1367]
      tunnel: w966 -> [w1362]
      tunnel: [w1361] -> w641
      frame #0 {
        # "Write Data"
        n180 = To Single Precision Float(number="Capacitance (uF)") -> (single precision float=w1356:sgl)
        n181 = To Variant(anything=w1356) -> (Variant=w1357:variant)
      }
      frame #1 {
        # "Resolve To TC"
        n182 = call <userlib>:"Resolve To TC Type.vi"("Handle"=w1367, "TypHdl"=w1368, "WData"=w1362, "error in"=w1369) -> ("Handle"=w1365:u32, "TypHdl"=w1366:u32, "bHasMatched"=w1361:bool, "ADSWData"=w1364:variant, "error out"=w1363:errorcluster)  [unwired: 7 in]
      }
    }
    n183 = flat-sequence {
      tunnel: w811 -> [w1328]
      tunnel: w810 -> [w1329]
      tunnel: w809 -> [w1330]
      tunnel: [w1330] -> w961
      tunnel: [w1329] -> w960
      tunnel: [w1328] -> w959
      tunnel: [w1327] -> w958
      tunnel: w701 -> [w1325]
      tunnel: [w1333] -> w596
      tunnel: [w1336] -> w805
      tunnel: [w1335] -> w806
      tunnel: [w1334] -> w769
      tunnel: w961 -> [w1339]
      tunnel: w960 -> [w1338]
      tunnel: w959 -> [w1337]
      tunnel: w958 -> [w1332]
      tunnel: [w1331] -> w645
      frame #0 {
        # "Write Data"
        n184 = To Long Integer(number=w1325) -> (32bit integer=w1326:i32)
        n185 = To Variant(anything=w1326) -> (Variant=w1327:variant)
      }
      frame #1 {
        # "Resolve To TC"
        n186 = call <userlib>:"Resolve To TC Type.vi"("Handle"=w1337, "TypHdl"=w1338, "WData"=w1332, "error in"=w1339) -> ("Handle"=w1335:u32, "TypHdl"=w1336:u32, "bHasMatched"=w1331:bool, "ADSWData"=w1334:variant, "error out"=w1333:errorcluster)  [unwired: 7 in]
      }
    }
    n187 = flat-sequence {
      tunnel: w823 -> [w1343]
      tunnel: w822 -> [w1344]
      tunnel: w821 -> [w1345]
      tunnel: [w1345] -> w965
      tunnel: [w1344] -> w964
      tunnel: [w1343] -> w963
      tunnel: [w1342] -> w962
      tunnel: [w1348] -> w599
      tunnel: [w1351] -> w817
      tunnel: [w1350] -> w818
      tunnel: [w1349] -> w770
      tunnel: w965 -> [w1354]
      tunnel: w964 -> [w1353]
      tunnel: w963 -> [w1352]
      tunnel: w962 -> [w1347]
      tunnel: [w1346] -> w643
      frame #0 {
        # "Write Data"
        n188 = To Long Integer(number="Target Charge Volt (V) - Min 1500V - TEMPORARY LIMIT 12kV") -> (32bit integer=w1341:i32)
        n189 = To Variant(anything=w1341) -> (Variant=w1342:variant)
      }
      frame #1 {
        # "Resolve To TC"
        n190 = call <userlib>:"Resolve To TC Type.vi"("Handle"=w1352, "TypHdl"=w1353, "WData"=w1347, "error in"=w1354) -> ("Handle"=w1350:u32, "TypHdl"=w1351:u32, "bHasMatched"=w1346:bool, "ADSWData"=w1349:variant, "error out"=w1348:errorcluster)  [unwired: 7 in]
      }
    }
    n191 = flat-sequence {
      tunnel: w799 -> [w1313]
      tunnel: w798 -> [w1314]
      tunnel: w797 -> [w1315]
      tunnel: [w1315] -> w957
      tunnel: [w1314] -> w956
      tunnel: [w1313] -> w955
      tunnel: [w1312] -> w954
      tunnel: [w1318] -> w593
      tunnel: [w1321] -> w793
      tunnel: [w1320] -> w794
      tunnel: [w1319] -> w768
      tunnel: w957 -> [w1324]
      tunnel: w956 -> [w1323]
      tunnel: w955 -> [w1322]
      tunnel: w954 -> [w1317]
      tunnel: [w1316] -> w647
      frame #0 {
        # "Write Data"
        n192 = To Word Integer(number="Hold Time Before Shot (seconds)") -> (16bit integer=w1311:i16)
        n193 = To Variant(anything=w1311) -> (Variant=w1312:variant)
      }
      frame #1 {
        # "Resolve To TC"
        n194 = call <userlib>:"Resolve To TC Type.vi"("Handle"=w1322, "TypHdl"=w1323, "WData"=w1317, "error in"=w1324) -> ("Handle"=w1320:u32, "TypHdl"=w1321:u32, "bHasMatched"=w1316:bool, "ADSWData"=w1319:variant, "error out"=w1318:errorcluster)  [unwired: 7 in]
      }
    }
    n195 = To Word Integer(number="Cap 1 Fault Temp (Cel)") -> (16bit integer=w437:i16)
    n196 = flat-sequence {
      tunnel: w847 -> [w1223]
      tunnel: w846 -> [w1224]
      tunnel: w845 -> [w1225]
      tunnel: [w1225] -> w933
      tunnel: [w1224] -> w932
      tunnel: [w1223] -> w931
      tunnel: [w1222] -> w930
      tunnel: [w1228] -> w604
      tunnel: [w1231] -> w841
      tunnel: [w1230] -> w842
      tunnel: [w1229] -> w772
      tunnel: w933 -> [w1234]
      tunnel: w932 -> [w1233]
      tunnel: w931 -> [w1232]
      tunnel: w930 -> [w1227]
      tunnel: [w1226] -> w640
      frame #0 {
        # "Write Data"
        n197 = And(x="CLEAR FAULT", y="CLEAR FAULT") -> (x .and. y?=w1221:bool)
        n198 = To Variant(anything=w1221) -> (Variant=w1222:variant)
      }
      frame #1 {
        # "Resolve To TC"
        n199 = call <userlib>:"Resolve To TC Type.vi"("Handle"=w1232, "TypHdl"=w1233, "WData"=w1227, "error in"=w1234) -> ("Handle"=w1230:u32, "TypHdl"=w1231:u32, "bHasMatched"=w1226:bool, "ADSWData"=w1229:variant, "error out"=w1228:errorcluster)  [unwired: 7 in]
      }
    }
    n200 = flat-sequence {
      tunnel: w895 -> [w1283]
      tunnel: w894 -> [w1284]
      tunnel: w893 -> [w1285]
      tunnel: [w1285] -> w949
      tunnel: [w1284] -> w948
      tunnel: [w1283] -> w947
      tunnel: [w1282] -> w946
      tunnel: [w1288] -> w616
      tunnel: [w1291] -> w889
      tunnel: [w1290] -> w890
      tunnel: [w1289] -> w776
      tunnel: w949 -> [w1294]
      tunnel: w948 -> [w1293]
      tunnel: w947 -> [w1292]
      tunnel: w946 -> [w1287]
      tunnel: [w1286] -> w632
      frame #0 {
        # "Write Data"
        n201 = And(x="Hold", y="Hold") -> (x .and. y?=w1281:bool)
        n202 = To Variant(anything=w1281) -> (Variant=w1282:variant)
      }
      frame #1 {
        # "Resolve To TC"
        n203 = call <userlib>:"Resolve To TC Type.vi"("Handle"=w1292, "TypHdl"=w1293, "WData"=w1287, "error in"=w1294) -> ("Handle"=w1290:u32, "TypHdl"=w1291:u32, "bHasMatched"=w1286:bool, "ADSWData"=w1289:variant, "error out"=w1288:errorcluster)  [unwired: 7 in]
      }
    }
    n204 = flat-sequence {
      tunnel: w871 -> [w1253]
      tunnel: w870 -> [w1254]
      tunnel: w869 -> [w1255]
      tunnel: [w1255] -> w941
      tunnel: [w1254] -> w940
      tunnel: [w1253] -> w939
      tunnel: [w1252] -> w938
      tunnel: [w1258] -> w610
      tunnel: [w1261] -> w865
      tunnel: [w1260] -> w866
      tunnel: [w1259] -> w774
      tunnel: w941 -> [w1264]
      tunnel: w940 -> [w1263]
      tunnel: w939 -> [w1262]
      tunnel: w938 -> [w1257]
      tunnel: [w1256] -> w636
      frame #0 {
        # "Write Data"
        n205 = And(x="Shot", y="Shot") -> (x .and. y?=w1251:bool)
        n206 = To Variant(anything=w1251) -> (Variant=w1252:variant)
      }
      frame #1 {
        # "Resolve To TC"
        n207 = call <userlib>:"Resolve To TC Type.vi"("Handle"=w1262, "TypHdl"=w1263, "WData"=w1257, "error in"=w1264) -> ("Handle"=w1260:u32, "TypHdl"=w1261:u32, "bHasMatched"=w1256:bool, "ADSWData"=w1259:variant, "error out"=w1258:errorcluster)  [unwired: 7 in]
      }
    }
    n208 = flat-sequence {
      tunnel: w903 -> [w1299]
      tunnel: [w1295] -> _
      tunnel: w901 -> [w1300]
      tunnel: [w1300] -> w953
      tunnel: [w1295] -> w952
      tunnel: [w1299] -> w951
      tunnel: [w1298] -> w950
      tunnel: w902 -> [w1295]
      tunnel: [w1303] -> w619
      tunnel: [w1306] -> w905
      tunnel: [w1305] -> w904
      tunnel: [w1304] -> w777
      tunnel: w953 -> [w1309]
      tunnel: w952 -> [w1308]
      tunnel: w951 -> [w1307]
      tunnel: w950 -> [w1302]
      tunnel: [w1301] -> w630
      frame #0 {
        # "Write Data"
        n209 = And(x="Manual/Auto", y="Manual/Auto") -> (x .and. y?=w1297:bool)
        n210 = To Variant(anything=w1297) -> (Variant=w1298:variant)
      }
      frame #1 {
        # "Resolve To TC"
        n211 = call <userlib>:"Resolve To TC Type.vi"("Handle"=w1307, "TypHdl"=w1308, "WData"=w1302, "error in"=w1309) -> ("Handle"=w1305:u32, "TypHdl"=w1306:u32, "bHasMatched"=w1301:bool, "ADSWData"=w1304:variant, "error out"=w1303:errorcluster)  [unwired: 7 in]
      }
    }
    n212 = flat-sequence {
      tunnel: w883 -> [w1268]
      tunnel: w882 -> [w1269]
      tunnel: w881 -> [w1270]
      tunnel: [w1270] -> w945
      tunnel: [w1269] -> w944
      tunnel: [w1268] -> w943
      tunnel: [w1267] -> w942
      tunnel: [w1273] -> w613
      tunnel: [w1276] -> w877
      tunnel: [w1275] -> w878
      tunnel: [w1274] -> w775
      tunnel: w945 -> [w1279]
      tunnel: w944 -> [w1278]
      tunnel: w943 -> [w1277]
      tunnel: w942 -> [w1272]
      tunnel: [w1271] -> w634
      frame #0 {
        # "Write Data"
        n213 = And(x="Charge", y="Charge") -> (x .and. y?=w1266:bool)
        n214 = To Variant(anything=w1266) -> (Variant=w1267:variant)
      }
      frame #1 {
        # "Resolve To TC"
        n215 = call <userlib>:"Resolve To TC Type.vi"("Handle"=w1277, "TypHdl"=w1278, "WData"=w1272, "error in"=w1279) -> ("Handle"=w1275:u32, "TypHdl"=w1276:u32, "bHasMatched"=w1271:bool, "ADSWData"=w1274:variant, "error out"=w1273:errorcluster)  [unwired: 7 in]
      }
    }
    n216 = flat-sequence {
      tunnel: w859 -> [w1238]
      tunnel: w858 -> [w1239]
      tunnel: w857 -> [w1240]
      tunnel: [w1240] -> w937
      tunnel: [w1239] -> w936
      tunnel: [w1238] -> w935
      tunnel: [w1237] -> w934
      tunnel: [w1243] -> w607
      tunnel: [w1246] -> w853
      tunnel: [w1245] -> w854
      tunnel: [w1244] -> w773
      tunnel: w937 -> [w1249]
      tunnel: w936 -> [w1248]
      tunnel: w935 -> [w1247]
      tunnel: w934 -> [w1242]
      tunnel: [w1241] -> w638
      frame #0 {
        # "Write Data"
        n217 = And(x="HV Switch Mode", y="HV Switch Mode") -> (x .and. y?=w1236:bool)
        n218 = To Variant(anything=w1236) -> (Variant=w1237:variant)
      }
      frame #1 {
        # "Resolve To TC"
        n219 = call <userlib>:"Resolve To TC Type.vi"("Handle"=w1247, "TypHdl"=w1248, "WData"=w1242, "error in"=w1249) -> ("Handle"=w1245:u32, "TypHdl"=w1246:u32, "bHasMatched"=w1241:bool, "ADSWData"=w1244:variant, "error out"=w1243:errorcluster)  [unwired: 7 in]
      }
    }
    n220 = flat-sequence {
      tunnel: w919 -> [w1184]
      tunnel: w918 -> [w1185]
      tunnel: w917 -> [w1186]
      tunnel: [w1186] -> w692
      tunnel: [w1185] -> w691
      tunnel: [w1184] -> w690
      tunnel: [w1183] -> w689
      tunnel: w692 -> [w1195]
      tunnel: w691 -> [w1194]
      tunnel: w690 -> [w1193]
      tunnel: w689 -> [w1188]
      tunnel: [w1189] -> w622
      tunnel: [w1192] -> w913
      tunnel: [w1191] -> w914
      tunnel: [w1190] -> w688
      tunnel: [w1187] -> w628
      frame #0 {
        # "Write Data"
        n221 = And(x="STOP", y="STOP") -> (x .and. y?=w1182:bool)
        n222 = To Variant(anything=w1182) -> (Variant=w1183:variant)
      }
      frame #1 {
        # "Resolve To TC"
        n223 = call <userlib>:"Resolve To TC Type.vi"("Handle"=w1193, "TypHdl"=w1194, "WData"=w1188, "error in"=w1195) -> ("Handle"=w1191:u32, "TypHdl"=w1192:u32, "bHasMatched"=w1187:bool, "ADSWData"=w1190:variant, "error out"=w1189:errorcluster)  [unwired: 7 in]
      }
    }
    n224 = flat-sequence {
      tunnel: w581 -> [w1131]
      tunnel: w580 -> [w1127]
      tunnel: w579 -> [w1132]
      tunnel: [w1132] -> w590
      tunnel: [w1127] -> w589
      tunnel: [w1131] -> w588
      tunnel: [w1130] -> w587
      tunnel: [w1135] -> w439
      tunnel: [w1138] -> w574
      tunnel: [w1137] -> w575
      tunnel: [w1136] -> w578
      tunnel: w590 -> [w1141]
      tunnel: w589 -> [w1140]
      tunnel: w588 -> [w1139]
      tunnel: w587 -> [w1134]
      tunnel: [w1133] -> w572
      frame #0 {
        # "Write Data"
        n225 = And(x="Reset Test Number", y="Reset Test Number") -> (x .and. y?=w1129:bool)
        n226 = To Variant(anything=w1129) -> (Variant=w1130:variant)
      }
      frame #1 {
        # "Resolve To TC"
        n227 = call <userlib>:"Resolve To TC Type.vi"("Handle"=w1139, "TypHdl"=w1140, "WData"=w1134, "error in"=w1141) -> ("Handle"=w1137:u32, "TypHdl"=w1138:u32, "bHasMatched"=w1133:bool, "ADSWData"=w1136:variant, "error out"=w1135:errorcluster)  [unwired: 7 in]
      }
    }
    n228 = flat-sequence {
      tunnel: w929 -> [w1150]
      tunnel: w928 -> [w1151]
      tunnel: w925 -> [w1152]
      tunnel: [w1152] -> w687
      tunnel: [w1151] -> w686
      tunnel: [w1150] -> w685
      tunnel: [w1149] -> w684
      tunnel: [w1147] -> _
      tunnel: [w1147] -> w683
      tunnel: w700 -> [w1147]
      tunnel: w699 -> [w1146]
      tunnel: [w1146] -> w682
      tunnel: w698 -> [w1145]
      tunnel: [w1145] -> w681
      tunnel: w697 -> [w1144]
      tunnel: [w1144] -> w680
      tunnel: w696 -> [w1143]
      tunnel: [w1143] -> w679
      tunnel: ["START"] -> w516
      tunnel: w687 -> [w1166]
      tunnel: w686 -> [w1165]
      tunnel: w685 -> [w1164]
      tunnel: w684 -> [w1159]
      tunnel: [w1160] -> w678
      tunnel: [w1163] -> w677
      tunnel: [w1162] -> w676
      tunnel: [w1161] -> w675
      tunnel: [w1158] -> w674
      tunnel: w683 -> [w1157]
      tunnel: [w1157] -> w673
      tunnel: w682 -> [w1156]
      tunnel: [w1156] -> w672
      tunnel: w681 -> [w1155]
      tunnel: [w1155] -> w671
      tunnel: w680 -> [w1154]
      tunnel: [w1154] -> w670
      tunnel: [w1153] -> w669
      tunnel: w679 -> [w1153]
      tunnel: [w1177] -> w652
      tunnel: [w1178] -> w927
      tunnel: [w1179] -> w926
      tunnel: [w1180] -> w625
      tunnel: w678 -> [w1180]
      tunnel: w677 -> [w1179]
      tunnel: w676 -> [w1178]
      tunnel: w675 -> [w1169]
      tunnel: w674 -> [w1177]
      tunnel: w673 -> [w1176]
      tunnel: w672 -> [w1175]
      tunnel: w671 -> [w1174]
      tunnel: w670 -> [w1173]
      tunnel: w669 -> [w1172]
      tunnel: [w1171] -> w695
      tunnel: [w1170] -> w694
      tunnel: [w1168] -> w626
      tunnel: [w1167] -> w667
      frame #0 {
        # "Write Data"
        n229 = And(x="START", y="START") -> (x .and. y?=w1148:bool)
        n230 = To Variant(anything=w1148) -> (Variant=w1149:variant)
      }
      frame #1 {
        # "Resolve To TC"
        n231 = call <userlib>:"Resolve To TC Type.vi"("Handle"=w1164, "TypHdl"=w1165, "WData"=w1159, "error in"=w1166) -> ("Handle"=w1162:u32, "TypHdl"=w1163:u32, "bHasMatched"=w1158:bool, "ADSWData"=w1161:variant, "error out"=w1160:errorcluster)  [unwired: 7 in]
      }
      frame #2 {
        # "Write"
        n232 = call <userlib>:"Send Writer-Request.vi"("Handle"=w1176, "SymbolName"=w1175, "WriterMode"=w1174, "WriteHandle"=w1173, "error constant"=w1172, "ADS Write Data"=w1169) -> ("Handle"=w1171:u32, "WriteHandle"=w1170:u32, "Write status?"=w1167:bool, "error IO"=w1168:errorcluster)  [unwired: 5 in, 1 out]
      }
    }
    n233 = To Variant(anything=w437) -> (Variant=w436:variant)
    n234 = call-poly <userlib>:"Write TypeResolved.vi"("Handle"=w417, "SymbolName"=w427, "WData"=w428, "error constant"=w426) -> ("Write Status?"=w422:bool, "Has Matched?"=w423:bool, "error out"=w425:errorcluster)  [unwired: 8 in, 1 out]
    n235 = call-poly <userlib>:"Write TypeResolved.vi"("Handle"=w417, "SymbolName"=w434, "WData"=w436, "error constant"=w435) -> ("Write Status?"=w431:bool, "Has Matched?"=w433:bool, "error out"=w432:errorcluster)  [unwired: 8 in, 1 out]
    n236 = To Single Precision Float(number="Duty Cycle") -> (single precision float=w475:sgl)
    n237 = And(x="Voltage Held by PSU", y="Voltage Held by PSU") -> (x .and. y?=w464:bool)
    n238 = And(x="Current Control", y="Current Control") -> (x .and. y?=w482:bool)
    n239 = To Variant(anything=w475) -> (Variant=w479:variant)
    n240 = And(x="Dump", y="Dump") -> (x .and. y?=w491:bool)
    n241 = To Variant(anything=w464) -> (Variant=w462:variant)
    n242 = To Variant(anything=w482) -> (Variant=w480:variant)
    n243 = To Variant(anything=w491) -> (Variant=w492:variant)
    n244 = call-poly <userlib>:"Write TypeResolved.vi"("Handle"=w417, "SymbolName"=w465, "WData"=w462, "error constant"=w461) -> ("Write Status?"=w454:bool, "Has Matched?"=w455:bool, "error out"=w460:errorcluster)  [unwired: 8 in, 1 out]
    n245 = flat-sequence {
      tunnel: w792 -> [w1497]
      tunnel: w791 -> [w1495]
      tunnel: w790 -> [w1493]
      tunnel: [w1496] -> w1004
      tunnel: [w1494] -> w1003
      tunnel: [w1492] -> w1002
      tunnel: [w1491] -> w1001
      tunnel: [w1490] -> w1000
      tunnel: [w1489] -> w999
      tunnel: [w1488] -> w998
      tunnel: [w1487] -> w997
      tunnel: [w1486] -> w996
      tunnel: [w1485] -> w995
      tunnel: [w1484] -> w994
      tunnel: w788 -> [w1483]
      tunnel: w787 -> [w1482]
      tunnel: w786 -> [w1481]
      tunnel: w785 -> [w1480]
      tunnel: w784 -> [w1479]
      tunnel: w783 -> [w1478]
      tunnel: [w1477] -> w993
      tunnel: [w1476] -> w992
      tunnel: [w1475] -> w991
      tunnel: [w1474] -> w990
      tunnel: [w1473] -> w989
      tunnel: [w1472] -> w988
      tunnel: [w1471] -> w987
      tunnel: [w1470] -> w986
      tunnel: [w1469] -> w985
      tunnel: [w1468] -> w984
      tunnel: [w1467] -> w983
      tunnel: [w1466] -> w982
      tunnel: [w1465] -> w981
      tunnel: [w1464] -> w980
      tunnel: [w1463] -> w979
      tunnel: [w1462] -> w978
      tunnel: [w1461] -> w977
      tunnel: [w1460] -> w976
      tunnel: [w1459] -> w975
      tunnel: [w1458] -> w974
      tunnel: [w1457] -> w973
      tunnel: [w1456] -> w972
      tunnel: [w1455] -> w971
      tunnel: [w1454] -> w970
      tunnel: w751 -> [w1453]
      tunnel: [w1452] -> w750
      tunnel: [w1451] -> w749
      tunnel: [w1450] -> w748
      tunnel: [w1449] -> w747
      tunnel: [w1448] -> w746
      tunnel: w744 -> [w1371]
      tunnel: [w1447] -> w743
      tunnel: w741 -> [w1446]
      tunnel: [w1445] -> w740
      tunnel: [w1444] -> w739
      tunnel: [w1443] -> w738
      tunnel: w737 -> [w1442]
      tunnel: w736 -> [w1441]
      tunnel: [w1440] -> w735
      tunnel: [w1439] -> w734
      tunnel: [w1438] -> w733
      tunnel: [w1437] -> w732
      tunnel: [w1436] -> w731
      tunnel: [w1435] -> w730
      tunnel: [w1434] -> w729
      tunnel: [w1433] -> w728
      tunnel: w720 -> [w1432]
      tunnel: w719 -> [w1431]
      tunnel: w718 -> [w1430]
      tunnel: [w1429] -> w717
      tunnel: [w1428] -> w716
      tunnel: [w1427] -> w715
      tunnel: [w1426] -> w714
      tunnel: [w1425] -> w713
      tunnel: [w1424] -> w712
      tunnel: [w1423] -> w711
      tunnel: [w1422] -> w710
      tunnel: [w1421] -> w709
      tunnel: [w1420] -> w708
      tunnel: [w1419] -> w707
      tunnel: [w1418] -> w706
      tunnel: [w1372] -> _
      tunnel: w693 -> [w1372]
      tunnel: [w1417] -> w566
      tunnel: [w1416] -> w565
      tunnel: [w1415] -> w564
      tunnel: w563 -> [w1414]
      tunnel: [w1413] -> w560
      tunnel: w559 -> [w1412]
      tunnel: [w1411] -> w558
      tunnel: [w1410] -> w557
      tunnel: [w1409] -> w556
      tunnel: [w1408] -> w555
      tunnel: w554 -> [w1407]
      tunnel: w553 -> [w1406]
      tunnel: w552 -> [w1405]
      tunnel: [w1404] -> w551
      tunnel: [w1403] -> w550
      tunnel: [w1402] -> w548
      tunnel: [w1401] -> w546
      tunnel: [w1400] -> w545
      tunnel: [w1399] -> w544
      tunnel: [w1398] -> w543
      tunnel: [w1397] -> w540
      tunnel: w539 -> [w1396]
      tunnel: [w1395] -> w538
      tunnel: [w1394] -> w537
      tunnel: [w1393] -> w536
      tunnel: w514 -> [w1392]
      tunnel: w513 -> [w1391]
      tunnel: [w1390] -> w512
      tunnel: [w1389] -> w511
      tunnel: [w1388] -> w510
      tunnel: [w1387] -> w509
      tunnel: [w1386] -> w508
      tunnel: [w1385] -> w507
      tunnel: w506 -> [w1384]
      tunnel: [w1383] -> w505
      tunnel: [w1382] -> w504
      tunnel: [w1381] -> w503
      tunnel: w489 -> [w1380]
      tunnel: [w1379] -> w488
      tunnel: [w1378] -> w487
      tunnel: [w1377] -> w486
      tunnel: [w1376] -> w449
      tunnel: [w1375] -> w448
      tunnel: w447 -> [w1374]
      tunnel: [w1373] -> w446
      tunnel: [w1370] -> w441
      tunnel: w1004 -> [w1703]
      tunnel: w1003 -> [w1716]
      tunnel: w1002 -> [_]
      tunnel: w1001 -> [w1702]
      tunnel: w1000 -> [w1701]
      tunnel: w999 -> [w1536]
      tunnel: [w1631] -> w789
      tunnel: w998 -> [w1715]
      tunnel: w997 -> [w1717]
      tunnel: w996 -> [w1719]
      tunnel: w995 -> [w1545]
      tunnel: w994 -> [_]
      tunnel: w993 -> [w1698]
      tunnel: w992 -> [w1713]
      tunnel: w991 -> [w1711]
      tunnel: w990 -> [w1709]
      tunnel: w989 -> [w1707]
      tunnel: w988 -> [w1705]
      tunnel: [w1644] -> w782
      tunnel: w987 -> [w1697]
      tunnel: w986 -> [w1696]
      tunnel: w985 -> [w1695]
      tunnel: w984 -> [w1694]
      tunnel: w983 -> [w1693]
      tunnel: w982 -> [w1692]
      tunnel: w981 -> [_]
      tunnel: w980 -> [w1534]
      tunnel: w979 -> [_]
      tunnel: w978 -> [w1532]
      tunnel: w977 -> [_]
      tunnel: w976 -> [w1530]
      tunnel: w975 -> [_]
      tunnel: w974 -> [w1528]
      tunnel: w973 -> [_]
      tunnel: w972 -> [w1526]
      tunnel: w971 -> [_]
      tunnel: w970 -> [w1524]
      tunnel: [w1646] -> w781
      tunnel: [w1648] -> w780
      tunnel: [w1650] -> w779
      tunnel: [w1652] -> w778
      tunnel: w750 -> [w1522]
      tunnel: w749 -> [w1683]
      tunnel: w748 -> [_]
      tunnel: w747 -> [w1615]
      tunnel: w746 -> [w1679]
      tunnel: [w1635] -> w745
      tunnel: w743 -> [w1682]
      tunnel: [w1633] -> w742
      tunnel: w740 -> [w1681]
      tunnel: w739 -> [w1500]
      tunnel: w738 -> [_]
      tunnel: w735 -> [w1677]
      tunnel: w734 -> [w1676]
      tunnel: w733 -> [w1673]
      tunnel: w732 -> [w1672]
      tunnel: w731 -> [w1671]
      tunnel: w730 -> [w1670]
      tunnel: w729 -> [_]
      tunnel: w728 -> [_]
      tunnel: [w1637] -> w727
      tunnel: [w1639] -> w726
      tunnel: [w1654] -> w723
      tunnel: [w1657] -> w722
      tunnel: [w1656] -> w721
      tunnel: w717 -> [w1668]
      tunnel: w716 -> [w1666]
      tunnel: w715 -> [w1664]
      tunnel: w714 -> [w1540]
      tunnel: w713 -> [w1538]
      tunnel: w712 -> [w1542]
      tunnel: w711 -> [w1663]
      tunnel: w710 -> [w1662]
      tunnel: w709 -> [w1661]
      tunnel: w708 -> [_]
      tunnel: w707 -> [_]
      tunnel: w706 -> [_]
      tunnel: [w1642] -> w705
      tunnel: [w1640] -> w704
      tunnel: [w1629] -> w703
      tunnel: [w1630] -> w411
      tunnel: [w1621] -> w591
      tunnel: [w1623] -> w567
      tunnel: w566 -> [w1544]
      tunnel: w565 -> [w1626]
      tunnel: w564 -> [_]
      tunnel: [w1624] -> w562
      tunnel: w560 -> [w1618]
      tunnel: w558 -> [w1613]
      tunnel: w557 -> [w1610]
      tunnel: w556 -> [w1608]
      tunnel: w555 -> [w1595]
      tunnel: w551 -> [w1520]
      tunnel: w550 -> [w1607]
      tunnel: [w1606] -> w549
      tunnel: w548 -> [w1605]
      tunnel: [w1604] -> w547
      tunnel: w546 -> [w1603]
      tunnel: w545 -> [w1516]
      tunnel: w544 -> [w1602]
      tunnel: w543 -> [w1514]
      tunnel: [w1601] -> w542
      tunnel: [w1600] -> w541
      tunnel: w540 -> [w1518]
      tunnel: [w1599] -> w523
      tunnel: [w1598] -> w521
      tunnel: [w1597] -> w531
      tunnel: w538 -> [w1590]
      tunnel: w537 -> [w1512]
      tunnel: w536 -> [w1593]
      tunnel: [w1592] -> w535
      tunnel: w512 -> [w1586]
      tunnel: w511 -> [w1510]
      tunnel: w510 -> [w1588]
      tunnel: w509 -> [w1587]
      tunnel: w508 -> [w1582]
      tunnel: w507 -> [w1508]
      tunnel: w505 -> [w1568]
      tunnel: w504 -> [w1506]
      tunnel: w503 -> [w1581]
      tunnel: [w1574] -> w502
      tunnel: [w1573] -> w501
      tunnel: [w1572] -> w500
      tunnel: [w1571] -> w499
      tunnel: w488 -> [w1549]
      tunnel: w487 -> [w1566]
      tunnel: w486 -> [w1504]
      tunnel: [w1565] -> w485
      tunnel: w449 -> [w1502]
      tunnel: w448 -> [w1550]
      tunnel: w446 -> [w1498]
      tunnel: [w1546] -> w445
      tunnel: w441 -> [_]
      frame #0 {
        # "Read and Resolve Data."
        # "Read/Resolve Symbol N"
        # "Read Data and Resolve Type"
        n246 = call-poly <userlib>:"Read TypeResolved.vi"("Handle"=w1372, "SymbolName"=w1441, "error constant"=w1371) -> ("Handle"=w1434:u32, "Read Status?"=w1439:bool, "RData"=w1435:variant, "error out"=w1438:errorcluster)  [unwired: 9 in]
        n247 = call-poly <userlib>:"Read TypeResolved.vi"("Handle"=w1372, "SymbolName"=w1442, "error constant"=w1371) -> ("Handle"=w1433:u32, "Read Status?"=w1440:bool, "RData"=w1436:variant, "error out"=w1437:errorcluster)  [unwired: 9 in]
        n248 = call-poly <userlib>:"Read TypeResolved.vi"("Handle"=w1372, "SymbolName"=w1495, "error constant"=w1371) -> ("Handle"=w1485:u32, "Read Status?"=w1487:bool, "RData"=w1491:variant, "error out"=w1496:errorcluster)  [unwired: 9 in]
        n249 = call-poly <userlib>:"Read TypeResolved.vi"("Handle"=w1372, "SymbolName"=w1446, "error constant"=w1371) -> ("Handle"=w1443:u32, "Read Status?"=w1445:bool, "RData"=w1444:variant, "error out"=w1448:errorcluster)  [unwired: 9 in]
        n250 = call-poly <userlib>:"Read TypeResolved.vi"("Handle"=w1372, "SymbolName"=w1497, "error constant"=w1371) -> ("Handle"=w1484:u32, "Read Status?"=w1486:bool, "RData"=w1490:variant, "error out"=w1447:errorcluster)  [unwired: 9 in]
        n251 = call-poly <userlib>:"Read TypeResolved.vi"("Handle"=w1372, "SymbolName"=w1374, "error constant"=w1371) -> ("Read Status?"=w1373:bool, "RData"=w1376:variant, "error out"=w1375:errorcluster)  [unwired: 9 in, 1 out]
        n252 = call-poly <userlib>:"Read TypeResolved.vi"("Handle"=w1372, "SymbolName"=w1493, "error constant"=w1371) -> ("Handle"=w1492:u32, "Read Status?"=w1488:bool, "RData"=w1489:variant, "error out"=w1494:errorcluster)  [unwired: 9 in]
        n253 = call-poly <userlib>:"Read TypeResolved.vi"("Handle"=w1372, "SymbolName"=w1483, "error constant"=w1371) -> ("Handle"=w1465:u32, "Read Status?"=w1472:bool, "RData"=w1464:variant, "error out"=w1471:errorcluster)  [unwired: 9 in]
        n254 = call-poly <userlib>:"Read TypeResolved.vi"("Handle"=w1372, "SymbolName"=w1384, "error constant"=w1371) -> ("Read Status?"=w1383:bool, "RData"=w1382:variant, "error out"=w1381:errorcluster)  [unwired: 9 in, 1 out]
        n255 = call-poly <userlib>:"Read TypeResolved.vi"("Handle"=w1372, "SymbolName"=w1380, "error constant"=w1371) -> ("Read Status?"=w1379:bool, "RData"=w1377:variant, "error out"=w1378:errorcluster)  [unwired: 9 in, 1 out]
        n256 = call-poly <userlib>:"Read TypeResolved.vi"("Handle"=w1372, "SymbolName"=w1481, "error constant"=w1371) -> ("Handle"=w1461:u32, "Read Status?"=w1474:bool, "RData"=w1460:variant, "error out"=w1469:errorcluster)  [unwired: 9 in]
        n257 = call-poly <userlib>:"Read TypeResolved.vi"("Handle"=w1372, "SymbolName"=w1479, "error constant"=w1371) -> ("Handle"=w1457:u32, "Read Status?"=w1476:bool, "RData"=w1456:variant, "error out"=w1467:errorcluster)  [unwired: 9 in]
        n258 = call-poly <userlib>:"Read TypeResolved.vi"("Handle"=w1372, "SymbolName"=w1396, "error constant"=w1371) -> ("Read Status?"=w1395:bool, "RData"=w1394:variant, "error out"=w1393:errorcluster)  [unwired: 9 in, 1 out]
        n259 = call-poly <userlib>:"Read TypeResolved.vi"("Handle"=w1372, "SymbolName"=w1392, "error constant"=w1371) -> ("Read Status?"=w1390:bool, "RData"=w1389:variant, "error out"=w1388:errorcluster)  [unwired: 9 in, 1 out]
        n260 = call-poly <userlib>:"Read TypeResolved.vi"("Handle"=w1372, "SymbolName"=w1391, "error constant"=w1371) -> ("Read Status?"=w1386:bool, "RData"=w1385:variant, "error out"=w1387:errorcluster)  [unwired: 9 in, 1 out]
        n261 = call-poly <userlib>:"Read TypeResolved.vi"("Handle"=w1372, "SymbolName"=w1482, "error constant"=w1371) -> ("Handle"=w1463:u32, "Read Status?"=w1473:bool, "RData"=w1462:variant, "error out"=w1470:errorcluster)  [unwired: 9 in]
        n262 = call-poly <userlib>:"Read TypeResolved.vi"("Handle"=w1372, "SymbolName"=w1480, "error constant"=w1371) -> ("Handle"=w1459:u32, "Read Status?"=w1475:bool, "RData"=w1458:variant, "error out"=w1468:errorcluster)  [unwired: 9 in]
        n263 = call-poly <userlib>:"Read TypeResolved.vi"("Handle"=w1372, "SymbolName"=w1478, "error constant"=w1371) -> ("Handle"=w1455:u32, "Read Status?"=w1477:bool, "RData"=w1454:variant, "error out"=w1466:errorcluster)  [unwired: 9 in]
        n264 = call-poly <userlib>:"Read TypeResolved.vi"("Handle"=w1372, "SymbolName"=w1453, "error constant"=w1371) -> ("Handle"=w1450:u32, "Read Status?"=w1449:bool, "RData"=w1452:variant, "error out"=w1451:errorcluster)  [unwired: 9 in]
        n265 = call-poly <userlib>:"Read TypeResolved.vi"("Handle"=w1372, "SymbolName"=w1412, "error constant"=w1371) -> ("Handle"=w1370:u32, "Read Status?"=w1411:bool, "RData"=w1404:variant, "error out"=w1403:errorcluster)  [unwired: 9 in]
        n266 = call-poly <userlib>:"Read TypeResolved.vi"("Handle"=w1372, "SymbolName"=w1407, "error constant"=w1371) -> ("Read Status?"=w1410:bool, "RData"=w1397:variant, "error out"=w1402:errorcluster)  [unwired: 9 in, 1 out]
        n267 = call-poly <userlib>:"Read TypeResolved.vi"("Handle"=w1372, "SymbolName"=w1405, "error constant"=w1371) -> ("Read Status?"=w1408:bool, "RData"=w1398:variant, "error out"=w1399:errorcluster)  [unwired: 9 in, 1 out]
        n268 = call-poly <userlib>:"Read TypeResolved.vi"("Handle"=w1372, "SymbolName"=w1406, "error constant"=w1371) -> ("Read Status?"=w1409:bool, "RData"=w1400:variant, "error out"=w1401:errorcluster)  [unwired: 9 in, 1 out]
        n269 = call-poly <userlib>:"Read TypeResolved.vi"("Handle"=w1372, "SymbolName"=w1432, "error constant"=w1371) -> ("Handle"=w1420:u32, "Read Status?"=w1429:bool, "RData"=w1425:variant, "error out"=w1421:errorcluster)  [unwired: 9 in]
        n270 = call-poly <userlib>:"Read TypeResolved.vi"("Handle"=w1372, "SymbolName"=w1431, "error constant"=w1371) -> ("Handle"=w1419:u32, "Read Status?"=w1428:bool, "RData"=w1426:variant, "error out"=w1422:errorcluster)  [unwired: 9 in]
        n271 = call-poly <userlib>:"Read TypeResolved.vi"("Handle"=w1372, "SymbolName"=w1414, "error constant"=w1371) -> ("Handle"=w1415:u32, "Read Status?"=w1413:bool, "RData"=w1417:variant, "error out"=w1416:errorcluster)  [unwired: 9 in]
        n272 = call-poly <userlib>:"Read TypeResolved.vi"("Handle"=w1372, "SymbolName"=w1430, "error constant"=w1371) -> ("Handle"=w1418:u32, "Read Status?"=w1427:bool, "RData"=w1424:variant, "error out"=w1423:errorcluster)  [unwired: 9 in]
      }
      frame #1 {
        # "Cast Symbol N to LabVIEW Type"
        # "Variant To Data"
        n273 = To Variant(anything=w1542) -> (Variant=w1541:variant)
        n274 = To Variant(anything=w1514) -> (Variant=w1513:variant)
        n275 = To Variant(anything=w1540) -> (Variant=w1539:variant)
        n276 = To Variant(anything=w1508) -> (Variant=w1507:variant)
        n277 = To Variant(anything=w1510) -> (Variant=w1509:variant)
        n278 = To Variant(anything=w1502) -> (Variant=w1501:variant)
        n279 = To Variant(anything=w1512) -> (Variant=w1511:variant)
        n280 = To Variant(anything=w1504) -> (Variant=w1503:variant)
        n281 = To Variant(anything=w1506) -> (Variant=w1505:variant)
        n282 = To Variant(anything=w1538) -> (Variant=w1537:variant)
        n283 = To Variant(anything=w1522) -> (Variant=w1521:variant)
        n284 = To Variant(anything=w1520) -> (Variant=w1519:variant)
        n285 = To Variant(anything=w1518) -> (Variant=w1517:variant)
        n286 = To Variant(anything=w1532) -> (Variant=w1531:variant)
        n287 = To Variant(anything=w1500) -> (Variant=w1499:variant)
        n288 = To Variant(anything=w1516) -> (Variant=w1515:variant)
        n289 = To Variant(anything=w1536) -> (Variant=w1535:variant)
        n290 = To Variant(anything=w1534) -> (Variant=w1533:variant)
        n291 = To Variant(anything=w1524) -> (Variant=w1523:variant)
        n292 = To Variant(anything=w1544) -> (Variant=w1543:variant)
        n293 = To Variant(anything=w1530) -> (Variant=w1529:variant)
        n294 = To Variant(anything=w1526) -> (Variant=w1525:variant)
        n295 = To Variant(anything=w1528) -> (Variant=w1527:variant)
        n296 = And(x=w1549, y=w1498) -> (x .and. y?=w1548:bool)
        n297 = Variant To Data(error in=w1550, Variant=w1501) -> (data=→"Test Interval (Sec)":i32, error out=w1546:errorcluster)  [unwired: 1 in]
        n298 = And(x=w1568, y=w1548) -> (x .and. y?=w1567:bool)
        n299 = And(x=w1582, y=w1567) -> (x .and. y?=w1583:bool)
        n300 = And(x=w1586, y=w1583) -> (x .and. y?=w1585:bool)
        n301 = And(x=w1590, y=w1585) -> (x .and. y?=w1589:bool)
        n302 = And(x=w1595, y=w1589) -> (x .and. y?=w1594:bool)
        n303 = And(x=w1608, y=w1594) -> (x .and. y?=w1609:bool)
        n304 = And(x=w1610, y=w1609) -> (x .and. y?=w1611:bool)
        n305 = And(x=w1613, y=w1611) -> (x .and. y?=w1612:bool)
        n306 = And(x=w1615, y=w1612) -> (x .and. y?=w1614:bool)
        n307 = And(x=w1698, y=w1614) -> (x .and. y?=w1714:bool)
        n308 = And(x=w1713, y=w1714) -> (x .and. y?=w1712:bool)
        n309 = And(x=w1711, y=w1712) -> (x .and. y?=w1710:bool)
        n310 = And(x=w1709, y=w1710) -> (x .and. y?=w1708:bool)
        n311 = And(x=w1707, y=w1708) -> (x .and. y?=w1706:bool)
        n312 = And(x=w1705, y=w1706) -> (x .and. y?=w1704:bool)
        n313 = And(x=w1715, y=w1704) -> (x .and. y?=w1669:bool)
        n314 = And(x=w1668, y=w1669) -> (x .and. y?=w1667:bool)
        n315 = And(x=w1666, y=w1667) -> (x .and. y?=w1665:bool)
        n316 = And(x=w1664, y=w1665) -> (x .and. y?=w1617:bool)
        n317 = And(x=w1618, y=w1617) -> (x .and. y?=w1616:bool)
        n318 = And(x=w1676, y=w1616) -> (x .and. y?=w1675:bool)
        n319 = And(x=w1677, y=w1675) -> (x .and. y?=w1674:bool)
        n320 = And(x=w1681, y=w1674) -> (x .and. y?=w1680:bool)
        n321 = And(x=w1719, y=w1680) -> (x .and. y?=w1718:bool)
        n322 = Variant To Data(error in=w1626, Variant=w1543) -> (data=→"Cap 1 Voltage (HVPS)":i16, error out=w1624:errorcluster)  [unwired: 1 in]
        n323 = Variant To Data(error in=w1697, Variant=w1533) -> (data=→"Discharge Fault":bool, error out=w1646:errorcluster)  [unwired: 1 in]
        n324 = Variant To Data(error in=w1716, Variant=w1535) -> (data=→"Charge Fault":bool, error out=w1644:errorcluster)  [unwired: 1 in]
        n325 = Variant To Data(error in=w1695, Variant=w1529) -> (data=→"Cap 1 Temp\nExceeded Fault":bool, error out=w1650:errorcluster)  [unwired: 1 in]
        n326 = And(x=w1717, y=w1718) -> (x .and. y?=→"Read Status":bool)
        n327 = Variant To Data(error in=w1696, Variant=w1531) -> (data=→"Hold Fault":bool, error out=w1648:errorcluster)  [unwired: 1 in]
        n328 = Variant To Data(error in=w1663, Variant=w1541) -> (data=→"Load Temperature":i16, error out=w1629:errorcluster)  [unwired: 1 in]
        n329 = Variant To Data(error in=w1694, Variant=w1527) -> (data=→"Ambient Temp\nExceeded Fault":bool, error out=w1652:errorcluster)  [unwired: 1 in]
        n330 = Variant To Data(error in=w1693, Variant=w1525) -> (data=→"PSU Fault":bool, error out=w1654:errorcluster)  [unwired: 1 in]
        n331 = Variant To Data(error in=w1692, Variant=w1523) -> (data=→"Control Sys Fault":bool, error out=w1656:errorcluster)  [unwired: 1 in]
        n332 = Variant To Data(error in=w1683, Variant=w1521) -> (data=→"test Running":bool, error out=w1657:errorcluster)  [unwired: 1 in]
        n333 = Variant To Data(error in=w1661, Variant=w1537) -> (data=→"Ambient Temp":i16, error out=w1642:errorcluster)  [unwired: 1 in]
        n334 = Variant To Data(error in=w1602, Variant=w1513) -> (data=w1597:bool, error out=w1600:errorcluster)  [unwired: 1 in]
        "Soft Exception" <- w1597
        n335 = Variant To Data(error in=w1593, Variant=w1511) -> (data=w1591:bool, error out=w1574:errorcluster)  [unwired: 1 in]
        "EOC" <- w1591
        n336 = Variant To Data(error in=w1662, Variant=w1539) -> (data=→"Soft Dump Temp":i16, error out=w1640:errorcluster)  [unwired: 1 in]
        n337 = Variant To Data(error in=w1607, Variant=w1519) -> (data=w1592:bool, error out=w1606:errorcluster)  [unwired: 1 in]
        "Softdump FB Fault" <- w1592
        n338 = Variant To Data(error in=w1603, Variant=w1515) -> (data=w1598:bool, error out=w1601:errorcluster)  [unwired: 1 in]
        "PSU HV FB Fault" <- w1598
        n339 = Variant To Data(error in=w1588, Variant=w1509) -> (data=w1562:bool, error out=w1573:errorcluster)  [unwired: 1 in]
        "SCR Ready" <- w1562
        n340 = Variant To Data(error in=w1587, Variant=w1507) -> (data=→"Maximum Test Number Reached":bool, error out=w1572:errorcluster)  [unwired: 1 in]
        n341 = Variant To Data(error in=w1605, Variant=w1517) -> (data=w1599:bool, error out=w1604:errorcluster)  [unwired: 1 in]
        "Charge FB Fault" <- w1599
        n342 = Variant To Data(error in=w1566, Variant=w1503) -> (data=w1563:bool, error out=w1565:errorcluster)  [unwired: 1 in]
        "Scope Trig" <- w1563
        n343 = Variant To Data(error in=w1679, Variant=w1499) -> (data=w1564:i16, error out=w1635:errorcluster)  [unwired: 1 in]
        "Process Step" <- w1564
        n344 = Variant To Data(error in=w1673, Variant=w1670) -> (data=→"Cap 1 Temperature":i16, error out=w1639:errorcluster)  [unwired: 1 in]
        n345 = Variant To Data(error in=w1672, Variant=w1671) -> (data=w1580:i16, error out=w1637:errorcluster)  [unwired: 1 in]
        "Cap 1 Voltage" <- w1580
        n346 = Variant To Data(error in=w1581, Variant=w1505) -> (data=w1570:i16, error out=w1571:errorcluster)  [unwired: 1 in]
        "Expected Voltage" <- w1570
        n347 = Variant To Data(error in=w1703, Variant=w1702) -> (data=→"Estimated Charge Time (seconds)":sgl, error out=w1631:errorcluster)  [unwired: 1 in]
        n348 = To Double Precision Float(number=w1580) -> (double precision float=→"Waveform Chart - Capacitor Voltage (Probe, abs(Volts))":dbl)
        n349 = Variant To Data(error in=w1682, Variant=w1701) -> (data=→"Shot Number":i16, error out=w1633:errorcluster)  [unwired: 1 in]
        n350 = case shown="True" "Log Temperature Data" {
          tunnel: [errorcluster {"status"=FALSE, "code"=0, "source"=""} ("error out") w1729] -> w1623
          frame False {
          }
          frame True {
            n351 = local read "Cap 1 Temperature"() -> (w1730:i16)
            n352 = local read "test Running"() -> (w1728:bool)
            n353 = call "Write To Measurement File2"("Signals"=w1730, "Enable"=w1728, "Filename"="Capacitor Temperature Data Log File Path (.xlsx)") -> ("error out"=w1729:errorcluster)  [unwired: 14 in, 2 out]
          }
        }
        n354 = case shown="2" w1564 {
          tunnel: ["Charge" "Current Controlled Charge" "Hold - Ready for Shot" "Hold - Cap Open Circuited" "Shot" "Wait" "Dump" "Error" "Wait"] -> w1678
          tunnel: [TRUE TRUE TRUE TRUE TRUE TRUE FALSE FALSE FALSE] -> w1560
          tunnel: [FALSE ("Reset") FALSE ("Reset") FALSE ("Reset") FALSE ("Reset") TRUE ("Reset") FALSE ("Reset") FALSE ("Reset") TRUE ("Reset") FALSE ("Reset")] -> _
          frame 1 {
          }
          frame 6 {
          }
          frame 2 {
          }
          frame 7 {
          }
          frame 3 {
          }
          frame 4 {
          }
          frame 5 {
          }
          frame 99 {
          }
          frame 0, Default {
          }
        }
        "Test State" <- w1678
        n355 = local write "Scope Trig"(w1563) -> ()
        n356 = local read "Cap 1 Voltage"() -> (w1552:i16)
        n357 = case shown="True" "Log Capacitor Voltage" {
          tunnel: [errorcluster {"status"=FALSE, "code"=0, "source"=""} ("error out") w1726] -> w1621
          tunnel: w1580 -> [_ w1725]
          tunnel: w1560 -> [_ w1724]
          frame False {
          }
          frame True {
            n358 = local read "test Running"() -> (w1721:bool)
            n359 = And(x=w1724, y=w1721) -> (x .and. y?=w1722:bool)
            n360 = call "Write To Measurement File"("Signals"=w1725, "Enable"=w1722, "Filename"="Capacitor Voltage Data Log File Path (.xlsx)") -> ("error out"=w1726:errorcluster)  [unwired: 14 in, 2 out]
          }
        }
        n361 = Not(x=w1591) -> (.not. x?=w1578:bool)
        n362 = To Double Precision Float(number=w1552) -> (double precision float=w1576:dbl)
        n363 = To Double Precision Float(number=w1570) -> (double precision float=w1569:dbl)
        n364 = Boolean To (0,1)(Boolean=w1578) -> (0, 1=→"EOC":i16)
        n365 = Or(x=w1656, y=w1657) -> (x .or. y?=w1655:bool)
        n366 = Or(x=w1654, y=w1655) -> (x .or. y?=w1653:bool)
        n367 = Or(x=w1652, y=w1653) -> (x .or. y?=w1651:bool)
        n368 = Or(x=w1650, y=w1651) -> (x .or. y?=w1649:bool)
        n369 = Or(x=w1648, y=w1649) -> (x .or. y?=w1647:bool)
        n370 = Or(x=w1646, y=w1647) -> (x .or. y?=w1645:bool)
        n371 = Or(x=w1644, y=w1645) -> (x .or. y?=w1643:bool)
        n372 = Or(x=w1642, y=w1643) -> (x .or. y?=w1641:bool)
        n373 = Or(x=w1640, y=w1641) -> (x .or. y?=w1628:bool)
        n374 = Or(x=w1629, y=w1628) -> (x .or. y?=w1622:bool)
        n375 = Boolean To (0,1)(Boolean=w1562) -> (0, 1=→"SCR FB":i16)
        n376 = Bundle(w1576, w1569) -> (→"Capacitor Voltage":cluster{dbl, dbl})  [unwired: 1 in]
        n377 = local write "Process Step"(w1564) -> ()
        n378 = local read "Scope Trig"() -> (w1555:bool)
        n379 = local read "Test Interval (Sec)"() -> (w1558:i32)
        n380 = Not(x=w1555) -> (.not. x?=w1554:bool)
        n381 = call "Elapsed Time"("Time Target (s)"=w1558, "Reset"=w1554) -> ("Elapsed Time Text"=w1557:string)  [unwired: 10 in, 7 out]
        n382 = String Subset(string=w1557, offset (0)=2) -> (substring=→"Time Since Last Shot":string)  [unwired: 1 in]
        n383 = Or(x=w1623, y=w1622) -> (x .or. y?=w1620:bool)
        n384 = Or(x=w1621, y=w1620) -> (x .or. y?=w1619:bool)
        n385 = Or(x=w1639, y=w1619) -> (x .or. y?=w1638:bool)
        n386 = Or(x=w1637, y=w1638) -> (x .or. y?=w1636:bool)
        n387 = Or(x=w1635, y=w1636) -> (x .or. y?=w1634:bool)
        n388 = Or(x=w1633, y=w1634) -> (x .or. y?=w1632:bool)
        n389 = Or(x=w1631, y=w1632) -> (x .or. y?=w1630:bool)
        "Internal TwinCAT Handle ID Maps" <- w1545
      }
    }
    n390 = call-poly <userlib>:"Write TypeResolved.vi"("Handle"=w417, "SymbolName"=w483, "WData"=w479, "error constant"=w461) -> ("Write Status?"=w453:bool, "Has Matched?"=w456:bool, "error out"=w477:errorcluster)  [unwired: 8 in, 1 out]
    n391 = call-poly <userlib>:"Write TypeResolved.vi"("Handle"=w417, "SymbolName"=w484, "WData"=w480, "error constant"=w461) -> ("Write Status?"=w452:bool, "Has Matched?"=w457:bool, "error out"=w478:errorcluster)  [unwired: 8 in, 1 out]
    n392 = call <userlib>:"Send Writer-Request.vi"("Handle"=w924, "SymbolName"=w923, "WriterMode"=w922, "WriteHandle"=w921, "error constant"=w920, "ADS Write Data"=w688) -> ("Handle"=w916:u32, "WriteHandle"=w915:u32, "Write status?"=w666:bool, "error IO"=w623:errorcluster)  [unwired: 5 in, 1 out]
    n393 = call-poly <userlib>:"Write TypeResolved.vi"("Handle"=w417, "SymbolName"=w498, "WData"=w492, "error constant"=w497) -> ("Handle"=w493:u32, "Write Status?"=w451:bool, "Has Matched?"=w459:bool, "error out"=w494:errorcluster)  [unwired: 8 in]
    n394 = call <userlib>:"Send Writer-Request.vi"("Handle"=w763, "SymbolName"=w762, "WriterMode"=w761, "WriteHandle"=w752, "error constant"=w760, "ADS Write Data"=w444) -> ("Handle"=w759:u32, "WriteHandle"=w758:u32, "Write status?"=w470:bool, "error IO"=w443:errorcluster)  [unwired: 5 in, 1 out]
    n395 = call <userlib>:"Send Writer-Request.vi"("Handle"=w840, "SymbolName"=w839, "WriterMode"=w838, "WriteHandle"=w837, "error constant"=w836, "ADS Write Data"=w771) -> ("Handle"=w832:u32, "WriteHandle"=w831:u32, "Write status?"=w474:bool, "error IO"=w603:errorcluster)  [unwired: 5 in, 1 out]
    n396 = call <userlib>:"Send Writer-Request.vi"("Handle"=w816, "SymbolName"=w815, "WriterMode"=w814, "WriteHandle"=w813, "error constant"=w812, "ADS Write Data"=w769) -> ("Handle"=w808:u32, "WriteHandle"=w807:u32, "Write status?"=w472:bool, "error IO"=w597:errorcluster)  [unwired: 5 in, 1 out]
    n397 = call <userlib>:"Send Writer-Request.vi"("Handle"=w828, "SymbolName"=w827, "WriterMode"=w826, "WriteHandle"=w825, "error constant"=w824, "ADS Write Data"=w770) -> ("Handle"=w820:u32, "WriteHandle"=w819:u32, "Write status?"=w473:bool, "error IO"=w600:errorcluster)  [unwired: 5 in, 1 out]
    n398 = call <userlib>:"Send Writer-Request.vi"("Handle"=w804, "SymbolName"=w803, "WriterMode"=w802, "WriteHandle"=w801, "error constant"=w800, "ADS Write Data"=w768) -> ("Handle"=w796:u32, "WriteHandle"=w795:u32, "Write status?"=w471:bool, "error IO"=w594:errorcluster)  [unwired: 5 in, 1 out]
    n399 = call <userlib>:"Send Writer-Request.vi"("Handle"=w912, "SymbolName"=w911, "WriterMode"=w910, "WriteHandle"=w908, "error constant"=w909, "ADS Write Data"=w777) -> ("Handle"=w907:u32, "WriteHandle"=w906:u32, "Write status?"=w654:bool, "error IO"=w620:errorcluster)  [unwired: 5 in, 1 out]
    n400 = call <userlib>:"Send Writer-Request.vi"("Handle"=w852, "SymbolName"=w851, "WriterMode"=w850, "WriteHandle"=w849, "error constant"=w848, "ADS Write Data"=w772) -> ("Handle"=w844:u32, "WriteHandle"=w843:u32, "Write status?"=w664:bool, "error IO"=w605:errorcluster)  [unwired: 5 in, 1 out]
    n401 = call <userlib>:"Send Writer-Request.vi"("Handle"=w900, "SymbolName"=w899, "WriterMode"=w898, "WriteHandle"=w897, "error constant"=w896, "ADS Write Data"=w776) -> ("Handle"=w892:u32, "WriteHandle"=w891:u32, "Write status?"=w656:bool, "error IO"=w617:errorcluster)  [unwired: 5 in, 1 out]
    n402 = call <userlib>:"Send Writer-Request.vi"("Handle"=w876, "SymbolName"=w875, "WriterMode"=w874, "WriteHandle"=w873, "error constant"=w872, "ADS Write Data"=w774) -> ("Handle"=w868:u32, "WriteHandle"=w867:u32, "Write status?"=w660:bool, "error IO"=w611:errorcluster)  [unwired: 5 in, 1 out]
    n403 = call <userlib>:"Send Writer-Request.vi"("Handle"=w888, "SymbolName"=w887, "WriterMode"=w886, "WriteHandle"=w885, "error constant"=w884, "ADS Write Data"=w775) -> ("Handle"=w880:u32, "WriteHandle"=w879:u32, "Write status?"=w658:bool, "error IO"=w614:errorcluster)  [unwired: 5 in, 1 out]
    n404 = call <userlib>:"Send Writer-Request.vi"("Handle"=w864, "SymbolName"=w863, "WriterMode"=w862, "WriteHandle"=w861, "error constant"=w860, "ADS Write Data"=w773) -> ("Handle"=w856:u32, "WriteHandle"=w855:u32, "Write status?"=w662:bool, "error IO"=w608:errorcluster)  [unwired: 5 in, 1 out]
    n405 = call <userlib>:"Send Writer-Request.vi"("Handle"=w586, "SymbolName"=w585, "WriterMode"=w584, "WriteHandle"=w583, "error constant"=w582, "ADS Write Data"=w578) -> ("Handle"=w577:u32, "WriteHandle"=w576:u32, "Write status?"=w570:bool, "error IO"=w440:errorcluster)  [unwired: 5 in, 1 out]
    n406 = Compound Arithmetic op=AND(w459, w457, w456, w455) -> (w458:bool)
    n407 = And(x=w433, y=w458) -> (x .and. y?=w495:bool)
    n408 = And(x=w423, y=w495) -> (x .and. y?=w568:bool)
    n409 = And(x=w650, y=w568) -> (x .and. y?=w649:bool)
    n410 = And(x=w413, y=w649) -> (x .and. y?=w648:bool)
    n411 = And(x=w647, y=w648) -> (x .and. y?=w646:bool)
    n412 = And(x=w645, y=w646) -> (x .and. y?=w644:bool)
    n413 = And(x=w643, y=w644) -> (x .and. y?=w642:bool)
    n414 = And(x=w641, y=w642) -> (x .and. y?=w408:bool)
    n415 = And(x=w572, y=w408) -> (x .and. y?=w573:bool)
    n416 = And(x=w640, y=w573) -> (x .and. y?=w639:bool)
    n417 = And(x=w638, y=w639) -> (x .and. y?=w637:bool)
    n418 = And(x=w636, y=w637) -> (x .and. y?=w635:bool)
    n419 = And(x=w634, y=w635) -> (x .and. y?=w633:bool)
    n420 = And(x=w632, y=w633) -> (x .and. y?=w631:bool)
    n421 = And(x=w630, y=w631) -> (x .and. y?=w629:bool)
    n422 = And(x=w628, y=w629) -> (x .and. y?=w627:bool)
    n423 = And(x=w652, y=w627) -> (x .and. y?=→"bHasMached":bool)
    n424 = Compound Arithmetic op=AND(w451, w452, w453, w454) -> (w450:bool)
    n425 = And(x=w431, y=w450) -> (x .and. y?=w496:bool)
    n426 = And(x=w422, y=w496) -> (x .and. y?=w467:bool)
    n427 = Compound Arithmetic op=AND(w474, w473, w472, w471, w412, w470) -> (w469:bool)
    n428 = Not(x=w469) -> (.not. x?=w468:bool)
    n429 = And(x=w468, y=w467) -> (x .and. y?=w466:bool)
    n430 = And(x=w570, y=w466) -> (x .and. y?=w571:bool)
    n431 = And(x=w664, y=w571) -> (x .and. y?=w663:bool)
    n432 = And(x=w662, y=w663) -> (x .and. y?=w661:bool)
    n433 = And(x=w660, y=w661) -> (x .and. y?=w659:bool)
    n434 = And(x=w658, y=w659) -> (x .and. y?=w657:bool)
    n435 = And(x=w656, y=w657) -> (x .and. y?=w655:bool)
    n436 = And(x=w654, y=w655) -> (x .and. y?=w653:bool)
    n437 = And(x=w666, y=w653) -> (x .and. y?=w665:bool)
    n438 = And(x=w667, y=w665) -> (x .and. y?=→"Write Status":bool)
    n439 = feedback #2(TRUE) -> (w518:bool)
    n440 = And(x=w518, y=w521) -> (x .and. y?=w520:bool)
    n441 = feedback #3(TRUE) -> (w528:bool)
    n442 = And(x=w528, y=w531) -> (x .and. y?=w530:bool)
    n443 = feedback #4(TRUE) -> (w532:bool)
    n444 = And(x=w532, y=w535) -> (x .and. y?=w534:bool)
    n445 = feedback #5(TRUE) -> (w524:bool)
    n446 = And(x=w524, y=w523) -> (x .and. y?=w525:bool)
    n447 = case shown="True" w525 {
      tunnel: [w1115 FALSE] -> w515
      tunnel: w516 -> [w1117 _]
      frame False {
        n448 = Or(x=w1117, y=FALSE) -> (x .or. y?=w1115:bool)
      }
      frame True {
        n449 = call "Charge relay error"() -> ()  [unwired: 10 in, 2 out]
      }
    }
    n450 = feedback-in #5(w515) -> ()
    n451 = case shown="True" w520 {
      tunnel: [w1113 FALSE] -> w519
      tunnel: w515 -> [w1111 _]
      frame False {
        n452 = Or(x=w1111, y=FALSE) -> (x .or. y?=w1113:bool)
      }
      frame True {
        n453 = call "PSU HV error"() -> ()  [unwired: 10 in, 2 out]
      }
    }
    n454 = feedback-in #2(w519) -> ()
    n455 = case shown="True" w534 {
      tunnel: [w1124 FALSE] -> w533
      tunnel: w516 -> [w1123 _]
      frame False {
        n456 = Or(x=w1123, y=FALSE) -> (x .or. y?=w1124:bool)
      }
      frame True {
        n457 = call "Softdump error"() -> ()  [unwired: 10 in, 2 out]
      }
    }
    n458 = feedback-in #4(w533) -> ()
    n459 = case shown="True" w530 {
      tunnel: [w1119 FALSE] -> w529
      tunnel: w515 -> [w1120 _]
      frame False {
        n460 = Or(x=w1120, y=FALSE) -> (x .or. y?=w1119:bool)
      }
      frame True {
        n461 = call "Soft Exception"() -> ()  [unwired: 10 in, 2 out]
      }
    }
    n462 = feedback-in #3(w529) -> ()
    n463 = Compound Arithmetic op=OR(w592, w626, w625) -> (w624:bool)
    n464 = Compound Arithmetic op=OR(w624, w623, w622) -> (w621:bool)
    n465 = Compound Arithmetic op=OR(w621, w620, w619) -> (w618:bool)
    n466 = Compound Arithmetic op=OR(w618, w617, w616) -> (w615:bool)
    n467 = Compound Arithmetic op=OR(w615, w614, w613) -> (w612:bool)
    n468 = Compound Arithmetic op=OR(w612, w611, w610) -> (w609:bool)
    n469 = Compound Arithmetic op=OR(w609, w608, w607) -> (w606:bool)
    n470 = Compound Arithmetic op=OR(w606, w605, w604) -> (w569:bool)
    n471 = Compound Arithmetic op=OR(w569, w440, w439) -> (w561:bool)
    n472 = Compound Arithmetic op=OR(w561) -> (w409:bool)
    n473 = Compound Arithmetic op=OR(w409, w603, w602) -> (w601:bool)
    n474 = Compound Arithmetic op=OR(w601, w600, w599) -> (w598:bool)
    n475 = Compound Arithmetic op=OR(w598, w597, w596) -> (w595:bool)
    n476 = Compound Arithmetic op=OR(w595, w594, w593) -> (w414:bool)
    n477 = Compound Arithmetic op=OR(w414, w443, w442) -> (w424:bool)
    n478 = Compound Arithmetic op=OR(w424, "EXIT HMI", w411) -> (w410:bool)
    "Stop Loops" <- w410
    n479 = property on="Stop Loops" class="Bool (strict)"("Val(Sgnl)"=w410) -> ()  [unwired: 2 in, 2 out]
    n480 = node-c288() -> ()  [unwired: 1 in, 1 out]
  }
  n481 = node-c288(w92) -> (w91:errorcluster)
  n482 = call <userlib>:"Release Writer.vi"("Handle"=w241, "WriteHandle"=w240, "error in (no error)"=w239) -> ("error out"=w235:errorcluster)  [unwired: 11 in, 1 out]
  n483 = call <userlib>:"Release Writer.vi"("Handle"=w203, "WriteHandle"=w202, "error in (no error)"=w201) -> ("error out"=w197:errorcluster)  [unwired: 11 in, 1 out]
  n484 = call <userlib>:"Release Type.vi"("Handle"=w238, "TypeHandle"=w237, "error in (no error)"=w236) -> ("error out"=w234:errorcluster)  [unwired: 11 in, 1 out]
  n485 = call <userlib>:"Release Writer.vi"("Handle"=w222, "WriteHandle"=w221, "error in (no error)"=w220) -> ("error out"=w216:errorcluster)  [unwired: 11 in, 1 out]
  n486 = call <userlib>:"Release Type.vi"("Handle"=w200, "TypeHandle"=w199, "error in (no error)"=w198) -> ("error out"=w196:errorcluster)  [unwired: 11 in, 1 out]
  n487 = call <userlib>:"Release Writer.vi"("Handle"=w184, "WriteHandle"=w183, "error in (no error)"=w182) -> ("error out"=w178:errorcluster)  [unwired: 11 in, 1 out]
  n488 = call <userlib>:"Release Type.vi"("Handle"=w219, "TypeHandle"=w218, "error in (no error)"=w217) -> ("error out"=w215:errorcluster)  [unwired: 11 in, 1 out]
  n489 = call <userlib>:"Release Type.vi"("Handle"=w181, "TypeHandle"=w180, "error in (no error)"=w179) -> ("error out"=w177:errorcluster)  [unwired: 11 in, 1 out]
  n490 = call <userlib>:"Release Writer.vi"("Handle"=w391, "WriteHandle"=w390, "error in (no error)"=w401) -> ("error out"=w110:errorcluster)  [unwired: 11 in, 1 out]
  n491 = call <userlib>:"Release Writer.vi"("Handle"=w260, "WriteHandle"=w259, "error in (no error)"=w258) -> ("error out"=w254:errorcluster)  [unwired: 11 in, 1 out]
  n492 = call <userlib>:"Release Writer.vi"("Handle"=w356, "WriteHandle"=w355, "error in (no error)"=w354) -> ("error out"=w362:errorcluster)  [unwired: 11 in, 1 out]
  n493 = call <userlib>:"Release Writer.vi"("Handle"=w336, "WriteHandle"=w335, "error in (no error)"=w334) -> ("error out"=w330:errorcluster)  [unwired: 11 in, 1 out]
  n494 = call <userlib>:"Release Writer.vi"("Handle"=w298, "WriteHandle"=w297, "error in (no error)"=w296) -> ("error out"=w292:errorcluster)  [unwired: 11 in, 1 out]
  n495 = call <userlib>:"Release Type.vi"("Handle"=w257, "TypeHandle"=w256, "error in (no error)"=w255) -> ("error out"=w253:errorcluster)  [unwired: 11 in, 1 out]
  n496 = call <userlib>:"Release Type.vi"("Handle"=w351, "TypeHandle"=w352, "error in (no error)"=w353) -> ("error out"=w363:errorcluster)  [unwired: 11 in, 1 out]
  n497 = call <userlib>:"Release Type.vi"("Handle"=w333, "TypeHandle"=w332, "error in (no error)"=w331) -> ("error out"=w329:errorcluster)  [unwired: 11 in, 1 out]
  n498 = call <userlib>:"Release Writer.vi"("Handle"=w317, "WriteHandle"=w316, "error in (no error)"=w315) -> ("error out"=w311:errorcluster)  [unwired: 11 in, 1 out]
  n499 = call <userlib>:"Release Type.vi"("Handle"=w295, "TypeHandle"=w294, "error in (no error)"=w293) -> ("error out"=w291:errorcluster)  [unwired: 11 in, 1 out]
  n500 = call <userlib>:"Release Writer.vi"("Handle"=w279, "WriteHandle"=w278, "error in (no error)"=w277) -> ("error out"=w273:errorcluster)  [unwired: 11 in, 1 out]
  n501 = call <userlib>:"Release Type.vi"("Handle"=w314, "TypeHandle"=w313, "error in (no error)"=w312) -> ("error out"=w310:errorcluster)  [unwired: 11 in, 1 out]
  n502 = call <userlib>:"Release Type.vi"("Handle"=w276, "TypeHandle"=w275, "error in (no error)"=w274) -> ("error out"=w272:errorcluster)  [unwired: 11 in, 1 out]
  n503 = call <userlib>:"Release Writer.vi"("Handle"=w374, "WriteHandle"=w373, "error in (no error)"=w372) -> ("error out"=w368:errorcluster)  [unwired: 11 in, 1 out]
  n504 = call <userlib>:"Release Writer.vi"("Handle"=w75, "WriteHandle"=w74, "error in (no error)"=w10) -> ("error out"=w89:errorcluster)  [unwired: 11 in, 1 out]
  n505 = call <userlib>:"Release Writer.vi"("Handle"=w12, "WriteHandle"=w146, "error in (no error)"=w15) -> ("Handle"=w4:u32, "error out"=w152:errorcluster)  [unwired: 11 in]
  n506 = call <userlib>:"Release Type.vi"("Handle"=w371, "TypeHandle"=w370, "error in (no error)"=w369) -> ("error out"=w367:errorcluster)  [unwired: 11 in, 1 out]
  n507 = call <userlib>:"Release Type.vi"("Handle"=w73, "TypeHandle"=w72, "error in (no error)"=w9) -> ("error out"=w88:errorcluster)  [unwired: 11 in, 1 out]
  n508 = call <userlib>:"Release Type.vi"("Handle"=w142, "TypeHandle"=w141, "error in (no error)"=w14) -> ("error out"=w151:errorcluster)  [unwired: 11 in, 1 out]
  n509 = call <userlib>:"Release Type.vi"("Handle"=w389, "TypeHandle"=w388, "error in (no error)"=w400) -> ("error out"=w111:errorcluster)  [unwired: 11 in, 1 out]
  n510 = Merge Errors(w235, w234) -> (w99:errorcluster)
  n511 = Merge Errors(w197, w196) -> (w97:errorcluster)
  n512 = Merge Errors(w216, w215) -> (w98:errorcluster)
  n513 = Merge Errors(w178, w177) -> (w96:errorcluster)
  n514 = Merge Errors(w362, w363) -> (w105:errorcluster)
  n515 = Merge Errors(w254, w253) -> (w100:errorcluster)
  n516 = Merge Errors(w330, w329) -> (w104:errorcluster)
  n517 = Merge Errors(w292, w291) -> (w102:errorcluster)
  n518 = Merge Errors(w311, w310) -> (w103:errorcluster)
  n519 = Merge Errors(w273, w272) -> (w101:errorcluster)
  n520 = Merge Errors(w368, w367) -> (w106:errorcluster)
  n521 = Merge Errors(w89, w88) -> (w87:errorcluster)
  n522 = Merge Errors(w152, w151) -> (w95:errorcluster)
  n523 = Merge Errors(w110, w111) -> (w109:errorcluster)
  n524 = Merge Errors(w43, w42, w41, w40, w32, w16) -> (w38:errorcluster)
  n525 = Merge Errors(w105, w104, w103, w102, w101, w100, w87) -> (w169:errorcluster)
  n526 = Merge Errors(w99, w98, w97, w96, w1, w95, w5, w7, w27, w26, w25, w21) -> (w168:errorcluster)
  n527 = Merge Errors(w121, w122, w123, w124, w125, w68, w67, w63, w64, w65, w66) -> (w112:errorcluster)
  n528 = Merge Errors(w90, w120, w119, w118, w117, w116, w115, w114, w54, w53, w52, w39, w38) -> (w113:errorcluster)
  n529 = Merge Errors(w112, w113) -> (w20:errorcluster)
  n530 = Merge Errors(w91, w109, w106, w169, w168, w20) -> (w107:errorcluster)
  n531 = call <userlib>:"Release.vi"("Handle"=w4, "error in (no error)"=w107) -> ("error out"=→"error out":errorcluster)  [unwired: 13 in]
